vi "T_MXC_control_PK_v1.0.vi"() -> ()   [LabVIEW 2016]
uses:
  Labview Drivers/lake_shore_372/Lake Shore 372/Lake Shore 372.lvlib
panel:
  in  "Output (0: sample heater)":u16(ring) items=["sample heater", "output 1 (warm-up heater) ", "output 2 (analog/still)"]
  in  "Heater Range (0: Off)":u16(ring) items=["Off", "31.6 uA", "100 uA", "316 uA", "1.00 mA", "3.16 mA", "10.0 mA", "31.6 mA", "100 mA"]
  in  "Manual Output (0.000%)":dbl min=-100.0 max=100.0 step=0.001 format="%.3f"
  in  "VISA resource name":refnum<visa-resource-name>="COM3"
  in  "Channel":i32=6
  out "Temperature (K)":dbl=4.98178 format="%#_13g"
  out "Time(s)":dbl=152.218 format="%#_13g"
  out "No. of data points collected":i32=3271
  in  "?":bool
  out "Temperature vs time":cluster{dbl, "Field Reading":dbl}[](graph)=[{0.061, "Field Reading"=5.86421}, {0.103, "Field Reading"=5.86421}, {0.153, "Field Reading"=5.86355}, {0.192, "Field Reading"=5.86355}, {0.254, "Field Reading"=5.86259}, {0.293, "Field Reading"=5.86259}, {0.353, "Field Reading"=5.8614}, {0.394, "Field Reading"=5.8614}, {0.454, "Field Reading"=5.85996}, {0.493, "Field Reading"=5.85996}, {0.549, "Field Reading"=5.85871}, {0.589, "Field Reading"=5.85871}, {0.649, "Field Reading"=5.85721}, {0.688, "Field Reading"=5.85721}, {0.748, "Field Reading"=5.85589}, {0.787, "Field Reading"=5.85589}, {0.826, "Field Reading"=5.8544}, {0.88, "Field Reading"=5.8544}, {0.921, "Field Reading"=5.85278}, {0.98, "Field Reading"=5.85278}, {1.019, "Field Reading"=5.85123}, {1.08, "Field Reading"=5.85123}, {1.121, "Field Reading"=5.84991}, {1.179, "Field Reading"=5.84991}, {1.219, "Field Reading"=5.84991}, {1.269, "Field Reading"=5.8489}, {1.308, "Field Reading"=5.8489}, {1.368, "Field Reading"=5.84782}, {1.405, "Field Reading"=5.84782}, {1.454, "Field Reading"=5.84692}, {1.494, "Field Reading"=5.84692}, {1.555, "Field Reading"=5.84602}, {1.593, "Field Reading"=5.84602}, {1.653, "Field Reading"=5.84537}, {1.694, "Field Reading"=5.84537}, {1.754, "Field Reading"=5.84465}, {1.793, "Field Reading"=5.84465}, {1.854, "Field Reading"=5.84417}, {1.895, "Field Reading"=5.84417}, {1.953, "Field Reading"=5.84351}, {1.994, "Field Reading"=5.84351}, {2.054, "Field Reading"=5.84267}, {2.093, "Field Reading"=5.84267}, {2.152, "Field Reading"=5.84154}, {2.191, "Field Reading"=5.84154}, {2.251, "Field Reading"=5.84022}, {2.29, "Field Reading"=5.84022}, {2.348, "Field Reading"=5.83897}, {2.389, "Field Reading"=5.83897}, {2.449, "Field Reading"=5.83789}, {2.487, "Field Reading"=5.83789}, {2.527, "Field Reading"=5.83693}, {2.58, "Field Reading"=5.83693}, {2.618, "Field Reading"=5.83693}, {2.669, "Field Reading"=5.83603}, {2.707, "Field Reading"=5.83603}, {2.768, "Field Reading"=5.83526}, {2.81, "Field Reading"=5.83526}, {2.867, "Field Reading"=5.83466}, {2.906, "Field Reading"=5.83466}, {2.953, "Field Reading"=5.83394}, {2.992, "Field Reading"=5.83394}, {3.053, "Field Reading"=5.83322}, {3.092, "Field Reading"=5.83322}, {3.153, "Field Reading"=5.83263}, {3.192, "Field Reading"=5.83263}, {3.251, "Field Reading"=5.83179}, {3.29, "Field Reading"=5.83179}, {3.348, "Field Reading"=5.83065}, {3.387, "Field Reading"=5.83065}, {3.425, "Field Reading"=5.82945}, {3.48, "Field Reading"=5.82945}, {3.52, "Field Reading"=5.82945}, {3.569, "Field Reading"=5.82844}, {3.608, "Field Reading"=5.82844}, {3.667, "Field Reading"=5.82718}, {3.707, "Field Reading"=5.82718}, {3.755, "Field Reading"=5.82598}, {3.793, "Field Reading"=5.82598}, {3.857, "Field Reading"=5.82491}, {3.895, "Field Reading"=5.82491}, {3.954, "Field Reading"=5.82365}, {3.992, "Field Reading"=5.82365}, {4.05, "Field Reading"=5.82228}, {4.091, "Field Reading"=5.82228}, {4.149, "Field Reading"=5.82108}, {4.19, "Field Reading"=5.82108}, {4.249, "Field Reading"=5.81988}, {4.288, "Field Reading"=5.81988}, {4.327, "Field Reading"=5.81863}, {4.38, "Field Reading"=5.81863}, {4.421, "Field Reading"=5.81773}, {4.483, "Field Reading"=5.81773}, {4.524, "Field Reading"=5.81677}, {4.583, "Field Reading"=5.81677}, {4.621, "Field Reading"=5.816}, {4.681, "Field Reading"=5.816}, {4.722, "Field Reading"=5.81522}, {4.78, "Field Reading"=5.81522}, {4.819, "Field Reading"=5.81522}, {4.869, "Field Reading"=5.8148}, {4.911, "Field Reading"=5.8148}, {4.968, "Field Reading"=5.81432}, {5.007, "Field Reading"=5.81432}, {5.07, "Field Reading"=5.81384}, {5.109, "Field Reading"=5.81384}, {5.168, "Field Reading"=5.81324}, {5.207, "Field Reading"=5.81324}, {5.269, "Field Reading"=5.81247}, {5.31, "Field Reading"=5.81247}, {5.367, "Field Reading"=5.81205}, {5.406, "Field Reading"=5.81205}, {5.455, "Field Reading"=5.81163}, {5.494, "Field Reading"=5.81163}, {5.555, "Field Reading"=5.81145}, {5.595, "Field Reading"=5.81145}, {5.655, "Field Reading"=5.81091}, {5.694, "Field Reading"=5.81091}, {5.753, "Field Reading"=5.81037}, {5.794, "Field Reading"=5.81037}, {5.852, "Field Reading"=5.80995}, {5.891, "Field Reading"=5.80995}, {5.95, "Field Reading"=5.80954}, {5.988, "Field Reading"=5.80954}, {6.026, "Field Reading"=5.80918}, {6.081, "Field Reading"=5.80918}, {6.12, "Field Reading"=5.80918}, {6.17, "Field Reading"=5.8084}, {6.21, "Field Reading"=5.8084}, {6.27, "Field Reading"=5.80756}, {6.308, "Field Reading"=5.80756}, {6.367, "Field Reading"=5.80654}, {6.406, "Field Reading"=5.80654}, {6.457, "Field Reading"=5.80541}, {6.496, "Field Reading"=5.80541}, {6.554, "Field Reading"=5.80433}, {6.593, "Field Reading"=5.80433}, {6.652, "Field Reading"=5.80331}, {6.691, "Field Reading"=5.80331}, {6.751, "Field Reading"=5.8023}, {6.793, "Field Reading"=5.8023}, {6.851, "Field Reading"=5.80116}, {6.892, "Field Reading"=5.80116}, {6.949, "Field Reading"=5.80026}, {6.987, "Field Reading"=5.80026}, {7.029, "Field Reading"=5.79913}, {7.082, "Field Reading"=5.79913}, {7.122, "Field Reading"=5.79829}, {7.182, "Field Reading"=5.79829}, {7.223, "Field Reading"=5.79781}, {7.283, "Field Reading"=5.79781}, {7.324, "Field Reading"=5.79739}, {7.383, "Field Reading"=5.79739}, {7.422, "Field Reading"=5.79715}, {7.483, "Field Reading"=5.79715}, {7.523, "Field Reading"=5.79662}, {7.584, "Field Reading"=5.79662}, {7.625, "Field Reading"=5.79638}, {7.681, "Field Reading"=5.79638}, {7.722, "Field Reading"=5.7959}, {7.782, "Field Reading"=5.7959}, {7.824, "Field Reading"=5.7956}, {7.882, "Field Reading"=5.7956}, {7.921, "Field Reading"=5.7956}, {7.969, "Field Reading"=5.7947}, {8.008, "Field Reading"=5.7947}, {8.069, "Field Reading"=5.79374}, {8.107, "Field Reading"=5.79374}, {8.168, "Field Reading"=5.79255}, {8.208, "Field Reading"=5.79255}, {8.256, "Field Reading"=5.79111}, {8.297, "Field Reading"=5.79111}, {8.354, "Field Reading"=5.78962}, {8.393, "Field Reading"=5.78962}, {8.451, "Field Reading"=5.78794}, {8.492, "Field Reading"=5.78794}, {8.549, "Field Reading"=5.78627}, {8.59, "Field Reading"=5.78627}, {8.651, "Field Reading"=5.78447}, {8.691, "Field Reading"=5.78447}, {8.749, "Field Reading"=5.78286}, {8.789, "Field Reading"=5.78286}, {8.827, "Field Reading"=5.7813}, {8.882, "Field Reading"=5.7813}, {8.921, "Field Reading"=5.7813}, {8.969, "Field Reading"=5.77993}, {9.008, "Field Reading"=5.77993}, {9.056, "Field Reading"=5.77861}, {9.095, "Field Reading"=5.77861}, {9.157, "Field Reading"=5.77753}, {9.196, "Field Reading"=5.77753}, {9.257, "Field Reading"=5.7764}, {9.3, "Field Reading"=5.7764}, {9.356, "Field Reading"=5.77544}, {9.395, "Field Reading"=5.77544}, {9.457, "Field Reading"=5.77418}, {9.498, "Field Reading"=5.77418}, {9.555, "Field Reading"=5.77287}, {9.595, "Field Reading"=5.77287}, {9.653, "Field Reading"=5.77137}, {9.695, "Field Reading"=5.77137}, {9.755, "Field Reading"=5.77018}, {9.794, "Field Reading"=5.77018}, {9.852, "Field Reading"=5.76886}, {9.89, "Field Reading"=5.76886}, {9.95, "Field Reading"=5.76736}, {9.99, "Field Reading"=5.76736}, {10.029, "Field Reading"=5.76599}, {10.084, "Field Reading"=5.76599}, {10.125, "Field Reading"=5.76455}, {10.182, "Field Reading"=5.76455}, {10.222, "Field Reading"=5.76455}, {10.271, "Field Reading"=5.76342}, {10.31, "Field Reading"=5.76342}, {10.369, "Field Reading"=5.76252}, {10.41, "Field Reading"=5.76252}, {10.47, "Field Reading"=5.76162}, {10.51, "Field Reading"=5.76162}, {10.569, "Field Reading"=5.76019}, {10.608, "Field Reading"=5.76019}, {10.67, "Field Reading"=5.75911}, {10.711, "Field Reading"=5.75911}, {10.77, "Field Reading"=5.75827}, {10.808, "Field Reading"=5.75827}, {10.856, "Field Reading"=5.75761}, {10.895, "Field Reading"=5.75761}, {10.955, "Field Reading"=5.75714}, {10.995, "Field Reading"=5.75714}, {11.056, "Field Reading"=5.75672}, {11.096, "Field Reading"=5.75672}, {11.155, "Field Reading"=5.75618}, {11.195, "Field Reading"=5.75618}, {11.253, "Field Reading"=5.75552}, {11.291, "Field Reading"=5.75552}, {11.351, "Field Reading"=5.75504}, {11.39, "Field Reading"=5.75504}, {11.429, "Field Reading"=5.75426}, {11.483, "Field Reading"=5.75426}, {11.524, "Field Reading"=5.75343}, {11.581, "Field Reading"=5.75343}, {11.621, "Field Reading"=5.75343}, {11.672, "Field Reading"=5.75235}, {11.711, "Field Reading"=5.75235}, {11.769, "Field Reading"=5.75121}, {11.809, "Field Reading"=5.75121}, {11.858, "Field Reading"=5.74996}, {11.899, "Field Reading"=5.74996}, {11.955, "Field Reading"=5.7487}, {11.996, "Field Reading"=5.7487}, {12.058, "Field Reading"=5.74757}, {12.098, "Field Reading"=5.74757}, {12.155, "Field Reading"=5.74643}, {12.196, "Field Reading"=5.74643}, {12.256, "Field Reading"=5.74565}, {12.296, "Field Reading"=5.74565}, {12.355, "Field Reading"=5.74463}, {12.394, "Field Reading"=5.74463}, {12.452, "Field Reading"=5.74374}, {12.491, "Field Reading"=5.74374}, {12.551, "Field Reading"=5.74266}, {12.592, "Field Reading"=5.74266}, {12.652, "Field Reading"=5.7417}, {12.692, "Field Reading"=5.7417}, {12.751, "Field Reading"=5.74087}, {12.79, "Field Reading"=5.74087}, {12.852, "Field Reading"=5.73991}, {12.89, "Field Reading"=5.73991}, {12.93, "Field Reading"=5.73877}, {12.985, "Field Reading"=5.73877}, {13.024, "Field Reading"=5.7374}, {13.087, "Field Reading"=5.7374}, {13.125, "Field Reading"=5.7362}, {13.184, "Field Reading"=5.7362}, {13.222, "Field Reading"=5.73464}, {13.283, "Field Reading"=5.73464}, {13.322, "Field Reading"=5.73464}, {13.37, "Field Reading"=5.73327}, {13.409, "Field Reading"=5.73327}, {13.457, "Field Reading"=5.73183}, {13.496, "Field Reading"=5.73183}, {13.553, "Field Reading"=5.7304}, {13.592, "Field Reading"=5.7304}, {13.651, "Field Reading"=5.72908}, {13.692, "Field Reading"=5.72908}, {13.751, "Field Reading"=5.72795}, {13.791, "Field Reading"=5.72795}, {13.829, "Field Reading"=5.72693}, {13.884, "Field Reading"=5.72693}, {13.926, "Field Reading"=5.72579}, {13.982, "Field Reading"=5.72579}, {14.021, "Field Reading"=5.72579}, {14.071, "Field Reading"=5.72501}, {14.111, "Field Reading"=5.72501}, {14.169, "Field Reading"=5.72388}, {14.207, "Field Reading"=5.72388}, {14.259, "Field Reading"=5.72256}, {14.298, "Field Reading"=5.72256}, {14.356, "Field Reading"=5.72113}, {14.398, "Field Reading"=5.72113}, {14.457, "Field Reading"=5.71951}, {14.495, "Field Reading"=5.71951}, {14.552, "Field Reading"=5.71778}, {14.591, "Field Reading"=5.71778}, {14.652, "Field Reading"=5.7158}, {14.693, "Field Reading"=5.7158}, {14.751, "Field Reading"=5.71401}, {14.79, "Field Reading"=5.71401}, {14.852, "Field Reading"=5.71209}, {14.89, "Field Reading"=5.71209}, {14.929, "Field Reading"=5.71078}, {14.985, "Field Reading"=5.71078}, {15.024, "Field Reading"=5.7093}, {15.083, "Field Reading"=5.7093}, {15.124, "Field Reading"=5.70789}, {15.183, "Field Reading"=5.70789}, {15.223, "Field Reading"=5.70657}, {15.283, "Field Reading"=5.70657}, {15.323, "Field Reading"=5.70541}, {15.385, "Field Reading"=5.70541}, {15.423, "Field Reading"=5.70448}, {15.486, "Field Reading"=5.70448}, {15.526, "Field Reading"=5.70358}, {15.582, "Field Reading"=5.70358}, {15.621, "Field Reading"=5.70358}, {15.672, "Field Reading"=5.70281}, {15.712, "Field Reading"=5.70281}, {15.77, "Field Reading"=5.70197}, {15.812, "Field Reading"=5.70197}, {15.87, "Field Reading"=5.70116}, {15.911, "Field Reading"=5.70116}, {15.97, "Field Reading"=5.70035}, {16.009, "Field Reading"=5.70035}, {16.058, "Field Reading"=5.69937}, {16.098, "Field Reading"=5.69937}, {16.156, "Field Reading"=5.69859}, {16.197, "Field Reading"=5.69859}, {16.255, "Field Reading"=5.69751}, {16.297, "Field Reading"=5.69751}, {16.358, "Field Reading"=5.69643}, {16.398, "Field Reading"=5.69643}, {16.458, "Field Reading"=5.6953}, {16.498, "Field Reading"=5.6953}, {16.556, "Field Reading"=5.69416}, {16.595, "Field Reading"=5.69416}, {16.655, "Field Reading"=5.69317}, {16.695, "Field Reading"=5.69317}, {16.752, "Field Reading"=5.69204}, {16.79, "Field Reading"=5.69204}, {16.829, "Field Reading"=5.69093}, {16.886, "Field Reading"=5.69093}, {16.925, "Field Reading"=5.68964}, {16.983, "Field Reading"=5.68964}, {17.022, "Field Reading"=5.68964}, {17.075, "Field Reading"=5.68845}, {17.115, "Field Reading"=5.68845}, {17.171, "Field Reading"=5.68743}, {17.21, "Field Reading"=5.68743}, {17.258, "Field Reading"=5.68647}, {17.299, "Field Reading"=5.68647}, {17.355, "Field Reading"=5.68513}, {17.395, "Field Reading"=5.68513}, {17.45, "Field Reading"=5.68399}, {17.489, "Field Reading"=5.68399}, {17.528, "Field Reading"=5.68327}, {17.583, "Field Reading"=5.68327}, {17.622, "Field Reading"=5.68327}, {17.669, "Field Reading"=5.68271}, {17.712, "Field Reading"=5.68271}, {17.769, "Field Reading"=5.68214}, {17.808, "Field Reading"=5.68214}, {17.856, "Field Reading"=5.68175}, {17.896, "Field Reading"=5.68175}, {17.952, "Field Reading"=5.68103}, {17.993, "Field Reading"=5.68103}, {18.031, "Field Reading"=5.68028}, {18.082, "Field Reading"=5.68028}, {18.122, "Field Reading"=5.68028}, {18.169, "Field Reading"=5.67986}, {18.208, "Field Reading"=5.67986}, {18.255, "Field Reading"=5.67956}, {18.296, "Field Reading"=5.67956}, {18.351, "Field Reading"=5.67912}, {18.389, "Field Reading"=5.67912}, {18.428, "Field Reading"=5.6787}, {18.484, "Field Reading"=5.6787}, {18.523, "Field Reading"=5.6787}, {18.571, "Field Reading"=5.6781}, {18.612, "Field Reading"=5.6781}, {18.669, "Field Reading"=5.6775}, {18.708, "Field Reading"=5.6775}, {18.755, "Field Reading"=5.67717}, {18.796, "Field Reading"=5.67717}, {18.853, "Field Reading"=5.67669}, {18.893, "Field Reading"=5.67669}, {18.95, "Field Reading"=5.67624}, {18.989, "Field Reading"=5.67624}, {19.03, "Field Reading"=5.67562}, {19.082, "Field Reading"=5.67562}, {19.123, "Field Reading"=5.67562}, {19.169, "Field Reading"=5.67481}, {19.208, "Field Reading"=5.67481}, {19.258, "Field Reading"=5.6737}, {19.297, "Field Reading"=5.6737}, {19.355, "Field Reading"=5.67254}, {19.393, "Field Reading"=5.67254}, {19.451, "Field Reading"=5.6711}, {19.491, "Field Reading"=5.6711}, {19.551, "Field Reading"=5.66972}, {19.589, "Field Reading"=5.66972}, {19.627, "Field Reading"=5.66847}, {19.683, "Field Reading"=5.66847}, {19.722, "Field Reading"=5.66847}, {19.77, "Field Reading"=5.66718}, {19.812, "Field Reading"=5.66718}, {19.868, "Field Reading"=5.6659}, {19.91, "Field Reading"=5.6659}, {19.957, "Field Reading"=5.66464}, {19.997, "Field Reading"=5.66464}, {20.056, "Field Reading"=5.66365}, {20.095, "Field Reading"=5.66365}, {20.15, "Field Reading"=5.66296}, {20.189, "Field Reading"=5.66296}, {20.227, "Field Reading"=5.66243}, {20.282, "Field Reading"=5.66243}, {20.321, "Field Reading"=5.66243}, {20.369, "Field Reading"=5.66192}, {20.41, "Field Reading"=5.66192}, {20.458, "Field Reading"=5.66132}, {20.496, "Field Reading"=5.66132}, {20.552, "Field Reading"=5.66066}, {20.59, "Field Reading"=5.66066}, {20.628, "Field Reading"=5.66021}, {20.683, "Field Reading"=5.66021}, {20.723, "Field Reading"=5.66021}, {20.77, "Field Reading"=5.65967}, {20.808, "Field Reading"=5.65967}, {20.856, "Field Reading"=5.65908}, {20.896, "Field Reading"=5.65908}, {20.952, "Field Reading"=5.65848}, {20.992, "Field Reading"=5.65848}, {21.032, "Field Reading"=5.65791}, {21.082, "Field Reading"=5.65791}, {21.121, "Field Reading"=5.65791}, {21.169, "Field Reading"=5.65737}, {21.207, "Field Reading"=5.65737}, {21.257, "Field Reading"=5.65683}, {21.296, "Field Reading"=5.65683}, {21.351, "Field Reading"=5.65626}, {21.392, "Field Reading"=5.65626}, {21.43, "Field Reading"=5.6557}, {21.483, "Field Reading"=5.6557}, {21.524, "Field Reading"=5.6557}, {21.57, "Field Reading"=5.65519}, {21.609, "Field Reading"=5.65519}, {21.657, "Field Reading"=5.65471}, {21.698, "Field Reading"=5.65471}, {21.756, "Field Reading"=5.65426}, {21.796, "Field Reading"=5.65426}, {21.853, "Field Reading"=5.65378}, {21.891, "Field Reading"=5.65378}, {21.929, "Field Reading"=5.65309}, {21.981, "Field Reading"=5.65309}, {22.021, "Field Reading"=5.65309}, {22.07, "Field Reading"=5.65259}, {22.109, "Field Reading"=5.65259}, {22.156, "Field Reading"=5.65205}, {22.196, "Field Reading"=5.65205}, {22.252, "Field Reading"=5.6513}, {22.292, "Field Reading"=5.6513}, {22.331, "Field Reading"=5.65034}, {22.382, "Field Reading"=5.65034}, {22.421, "Field Reading"=5.65034}, {22.47, "Field Reading"=5.64926}, {22.508, "Field Reading"=5.64926}, {22.556, "Field Reading"=5.64825}, {22.594, "Field Reading"=5.64825}, {22.651, "Field Reading"=5.6472}, {22.691, "Field Reading"=5.6472}, {22.73, "Field Reading"=5.64618}, {22.781, "Field Reading"=5.64618}, {22.82, "Field Reading"=5.64618}, {22.87, "Field Reading"=5.64526}, {22.908, "Field Reading"=5.64526}, {22.956, "Field Reading"=5.64442}, {22.994, "Field Reading"=5.64442}, {23.052, "Field Reading"=5.64379}, {23.093, "Field Reading"=5.64379}, {23.151, "Field Reading"=5.64316}, {23.191, "Field Reading"=5.64316}, {23.231, "Field Reading"=5.6428}, {23.283, "Field Reading"=5.6428}, {23.323, "Field Reading"=5.6428}, {23.37, "Field Reading"=5.64242}, {23.409, "Field Reading"=5.64242}, {23.457, "Field Reading"=5.64206}, {23.496, "Field Reading"=5.64206}, {23.551, "Field Reading"=5.64158}, {23.592, "Field Reading"=5.64158}, {23.652, "Field Reading"=5.6411}, {23.691, "Field Reading"=5.6411}, {23.73, "Field Reading"=5.64071}, {23.781, "Field Reading"=5.64071}, {23.821, "Field Reading"=5.64071}, {23.87, "Field Reading"=5.64032}, {23.908, "Field Reading"=5.64032}, {23.957, "Field Reading"=5.6402}, {23.998, "Field Reading"=5.6402}, {24.058, "Field Reading"=5.64017}, {24.098, "Field Reading"=5.64017}, {24.157, "Field Reading"=5.63996}, {24.197, "Field Reading"=5.63996}, {24.253, "Field Reading"=5.63948}, {24.293, "Field Reading"=5.63948}, {24.332, "Field Reading"=5.63933}, {24.384, "Field Reading"=5.63933}, {24.422, "Field Reading"=5.63933}, {24.471, "Field Reading"=5.63883}, {24.511, "Field Reading"=5.63883}, {24.556, "Field Reading"=5.6382}, {24.597, "Field Reading"=5.6382}, {24.654, "Field Reading"=5.63715}, {24.695, "Field Reading"=5.63715}, {24.751, "Field Reading"=5.63604}, {24.79, "Field Reading"=5.63604}, {24.828, "Field Reading"=5.63464}, {24.883, "Field Reading"=5.63464}, {24.922, "Field Reading"=5.63464}, {24.97, "Field Reading"=5.63332}, {25.012, "Field Reading"=5.63332}, {25.059, "Field Reading"=5.63231}, {25.099, "Field Reading"=5.63231}, {25.153, "Field Reading"=5.63114}, {25.195, "Field Reading"=5.63114}, {25.252, "Field Reading"=5.63}, {25.292, "Field Reading"=5.63}, {25.333, "Field Reading"=5.62872}, {25.382, "Field Reading"=5.62872}, {25.422, "Field Reading"=5.62872}, {25.471, "Field Reading"=5.62752}, {25.511, "Field Reading"=5.62752}, {25.557, "Field Reading"=5.62626}, {25.595, "Field Reading"=5.62626}, {25.652, "Field Reading"=5.62501}, {25.691, "Field Reading"=5.62501}, {25.731, "Field Reading"=5.62354}, {25.787, "Field Reading"=5.62354}, {25.828, "Field Reading"=5.62205}, {25.883, "Field Reading"=5.62205}, {25.923, "Field Reading"=5.62205}, {25.97, "Field Reading"=5.62049}, {26.008, "Field Reading"=5.62049}, {26.057, "Field Reading"=5.61899}, {26.097, "Field Reading"=5.61899}, {26.153, "Field Reading"=5.61756}, {26.192, "Field Reading"=5.61756}, {26.233, "Field Reading"=5.61663}, {26.284, "Field Reading"=5.61663}, {26.323, "Field Reading"=5.61663}, {26.371, "Field Reading"=5.6157}, {26.41, "Field Reading"=5.6157}, {26.459, "Field Reading"=5.61481}, {26.499, "Field Reading"=5.61481}, {26.554, "Field Reading"=5.61379}, {26.592, "Field Reading"=5.61379}, {26.632, "Field Reading"=5.61271}, {26.685, "Field Reading"=5.61271}, {26.724, "Field Reading"=5.61271}, {26.771, "Field Reading"=5.61152}, {26.812, "Field Reading"=5.61152}, {26.858, "Field Reading"=5.61032}, {26.899, "Field Reading"=5.61032}, {26.953, "Field Reading"=5.60906}, {26.992, "Field Reading"=5.60906}, {27.032, "Field Reading"=5.60745}, {27.086, "Field Reading"=5.60745}, {27.125, "Field Reading"=5.60745}, {27.172, "Field Reading"=5.60565}, {27.212, "Field Reading"=5.60565}, {27.258, "Field Reading"=5.60404}, {27.296, "Field Reading"=5.60404}, {27.353, "Field Reading"=5.6026}, {27.393, "Field Reading"=5.6026}, {27.453, "Field Reading"=5.60114}, {27.492, "Field Reading"=5.60114}, {27.531, "Field Reading"=5.59988}, {27.586, "Field Reading"=5.59988}, {27.625, "Field Reading"=5.59988}, {27.673, "Field Reading"=5.59857}, {27.715, "Field Reading"=5.59857}, {27.771, "Field Reading"=5.59725}, {27.812, "Field Reading"=5.59725}, {27.859, "Field Reading"=5.59599}, {27.897, "Field Reading"=5.59599}, {27.954, "Field Reading"=5.59498}, {27.992, "Field Reading"=5.59498}, {28.033, "Field Reading"=5.59387}, {28.086, "Field Reading"=5.59387}, {28.124, "Field Reading"=5.59387}, {28.171, "Field Reading"=5.59267}, {28.211, "Field Reading"=5.59267}, {28.258, "Field Reading"=5.59157}, {28.296, "Field Reading"=5.59157}, {28.352, "Field Reading"=5.59046}, {28.393, "Field Reading"=5.59046}, {28.432, "Field Reading"=5.58941}, {28.485, "Field Reading"=5.58941}, {28.523, "Field Reading"=5.58941}, {28.57, "Field Reading"=5.58854}, {28.611, "Field Reading"=5.58854}, {28.659, "Field Reading"=5.58768}, {28.699, "Field Reading"=5.58768}, {28.754, "Field Reading"=5.58663}, {28.793, "Field Reading"=5.58663}, {28.831, "Field Reading"=5.58558}, {28.885, "Field Reading"=5.58558}, {28.926, "Field Reading"=5.58558}, {28.971, "Field Reading"=5.58487}, {29.01, "Field Reading"=5.58487}, {29.06, "Field Reading"=5.58412}, {29.099, "Field Reading"=5.58412}, {29.155, "Field Reading"=5.58337}, {29.196, "Field Reading"=5.58337}, {29.254, "Field Reading"=5.5828}, {29.293, "Field Reading"=5.5828}, {29.332, "Field Reading"=5.5822}, {29.384, "Field Reading"=5.5822}, {29.423, "Field Reading"=5.5822}, {29.471, "Field Reading"=5.58184}, {29.51, "Field Reading"=5.58184}, {29.558, "Field Reading"=5.58149}, {29.597, "Field Reading"=5.58149}, {29.654, "Field Reading"=5.58119}, {29.691, "Field Reading"=5.58119}, {29.732, "Field Reading"=5.58065}, {29.786, "Field Reading"=5.58065}, {29.824, "Field Reading"=5.58065}, {29.872, "Field Reading"=5.58008}, {29.911, "Field Reading"=5.58008}, {29.957, "Field Reading"=5.5796}, {29.998, "Field Reading"=5.5796}, {30.054, "Field Reading"=5.57903}, {30.093, "Field Reading"=5.57903}, {30.133, "Field Reading"=5.57829}, {30.184, "Field Reading"=5.57829}, {30.223, "Field Reading"=5.57829}, {30.272, "Field Reading"=5.57736}, {30.312, "Field Reading"=5.57736}, {30.358, "Field Reading"=5.57637}, {30.397, "Field Reading"=5.57637}, {30.454, "Field Reading"=5.57532}, {30.493, "Field Reading"=5.57532}, {30.53, "Field Reading"=5.57434}, {30.586, "Field Reading"=5.57434}, {30.625, "Field Reading"=5.57434}, {30.674, "Field Reading"=5.57332}, {30.715, "Field Reading"=5.57332}, {30.771, "Field Reading"=5.57212}, {30.811, "Field Reading"=5.57212}, {30.859, "Field Reading"=5.57072}, {30.897, "Field Reading"=5.57072}, {30.953, "Field Reading"=5.5694}, {30.993, "Field Reading"=5.5694}, {31.031, "Field Reading"=5.56785}, {31.086, "Field Reading"=5.56785}, {31.127, "Field Reading"=5.56647}, {31.185, "Field Reading"=5.56647}, {31.226, "Field Reading"=5.56647}, {31.274, "Field Reading"=5.56521}, {31.313, "Field Reading"=5.56521}, {31.371, "Field Reading"=5.5639}, {31.41, "Field Reading"=5.5639}, {31.46, "Field Reading"=5.56276}, {31.5, "Field Reading"=5.56276}, {31.555, "Field Reading"=5.56168}, {31.594, "Field Reading"=5.56168}, {31.633, "Field Reading"=5.56088}, {31.686, "Field Reading"=5.56088}, {31.726, "Field Reading"=5.56088}, {31.772, "Field Reading"=5.56004}, {31.813, "Field Reading"=5.56004}, {31.859, "Field Reading"=5.55935}, {31.9, "Field Reading"=5.55935}, {31.954, "Field Reading"=5.55875}, {31.992, "Field Reading"=5.55875}, {32.032, "Field Reading"=5.5578}, {32.085, "Field Reading"=5.5578}, {32.124, "Field Reading"=5.5578}, {32.171, "Field Reading"=5.55696}, {32.211, "Field Reading"=5.55696}, {32.259, "Field Reading"=5.55618}, {32.297, "Field Reading"=5.55618}, {32.353, "Field Reading"=5.55552}, {32.391, "Field Reading"=5.55552}, {32.43, "Field Reading"=5.55486}, {32.485, "Field Reading"=5.55486}, {32.525, "Field Reading"=5.55486}, {32.571, "Field Reading"=5.55427}, {32.613, "Field Reading"=5.55427}, {32.66, "Field Reading"=5.55391}, {32.699, "Field Reading"=5.55391}, {32.754, "Field Reading"=5.5537}, {32.793, "Field Reading"=5.5537}, {32.831, "Field Reading"=5.55367}, {32.886, "Field Reading"=5.55367}, {32.924, "Field Reading"=5.55367}, {32.973, "Field Reading"=5.55352}, {33.013, "Field Reading"=5.55352}, {33.06, "Field Reading"=5.55322}, {33.098, "Field Reading"=5.55322}, {33.154, "Field Reading"=5.55295}, {33.193, "Field Reading"=5.55295}, {33.232, "Field Reading"=5.55229}, {33.286, "Field Reading"=5.55229}, {33.327, "Field Reading"=5.55157}, {33.385, "Field Reading"=5.55157}, {33.423, "Field Reading"=5.55157}, {33.473, "Field Reading"=5.55071}, {33.513, "Field Reading"=5.55071}, {33.558, "Field Reading"=5.5499}, {33.598, "Field Reading"=5.5499}, {33.655, "Field Reading"=5.549}, {33.693, "Field Reading"=5.549}, {33.734, "Field Reading"=5.54831}, {33.784, "Field Reading"=5.54831}, {33.824, "Field Reading"=5.54831}, {33.874, "Field Reading"=5.54781}, {33.913, "Field Reading"=5.54781}, {33.959, "Field Reading"=5.54739}, {33.997, "Field Reading"=5.54739}, {34.055, "Field Reading"=5.54718}, {34.094, "Field Reading"=5.54718}, {34.134, "Field Reading"=5.54697}, {34.187, "Field Reading"=5.54697}, {34.227, "Field Reading"=5.54697}, {34.274, "Field Reading"=5.54673}, {34.315, "Field Reading"=5.54673}, {34.359, "Field Reading"=5.54619}, {34.399, "Field Reading"=5.54619}, {34.456, "Field Reading"=5.5458}, {34.496, "Field Reading"=5.5458}, {34.535, "Field Reading"=5.54526}, {34.585, "Field Reading"=5.54526}, {34.625, "Field Reading"=5.54526}, {34.675, "Field Reading"=5.54452}, {34.713, "Field Reading"=5.54452}, {34.759, "Field Reading"=5.54377}, {34.797, "Field Reading"=5.54377}, {34.855, "Field Reading"=5.54302}, {34.895, "Field Reading"=5.54302}, {34.954, "Field Reading"=5.54218}, {34.992, "Field Reading"=5.54218}, {35.032, "Field Reading"=5.54138}, {35.086, "Field Reading"=5.54138}, {35.125, "Field Reading"=5.54138}, {35.172, "Field Reading"=5.54075}, {35.211, "Field Reading"=5.54075}, {35.26, "Field Reading"=5.54024}, {35.299, "Field Reading"=5.54024}, {35.355, "Field Reading"=5.53966}, {35.394, "Field Reading"=5.53966}, {35.434, "Field Reading"=5.5391}, {35.486, "Field Reading"=5.5391}, {35.525, "Field Reading"=5.5391}, {35.572, "Field Reading"=5.53832}, {35.612, "Field Reading"=5.53832}, {35.659, "Field Reading"=5.53776}, {35.699, "Field Reading"=5.53776}, {35.754, "Field Reading"=5.53731}, {35.793, "Field Reading"=5.53731}, {35.832, "Field Reading"=5.53686}, {35.886, "Field Reading"=5.53686}, {35.925, "Field Reading"=5.53686}, {35.972, "Field Reading"=5.5363}, {36.011, "Field Reading"=5.5363}, {36.06, "Field Reading"=5.53557}, {36.1, "Field Reading"=5.53557}, {36.156, "Field Reading"=5.53495}, {36.196, "Field Reading"=5.53495}, {36.234, "Field Reading"=5.53422}, {36.286, "Field Reading"=5.53422}, {36.327, "Field Reading"=5.53422}, {36.374, "Field Reading"=5.53344}, {36.415, "Field Reading"=5.53344}, {36.474, "Field Reading"=5.53248}, {36.515, "Field Reading"=5.53248}, {36.56, "Field Reading"=5.53164}, {36.598, "Field Reading"=5.53164}, {36.655, "Field Reading"=5.53052}, {36.696, "Field Reading"=5.53052}, {36.755, "Field Reading"=5.52956}, {36.793, "Field Reading"=5.52956}, {36.832, "Field Reading"=5.52861}, {36.887, "Field Reading"=5.52861}, {36.926, "Field Reading"=5.52861}, {36.974, "Field Reading"=5.52755}, {37.012, "Field Reading"=5.52755}, {37.061, "Field Reading"=5.52654}, {37.099, "Field Reading"=5.52654}, {37.155, "Field Reading"=5.52581}, {37.195, "Field Reading"=5.52581}, {37.235, "Field Reading"=5.52508}, {37.287, "Field Reading"=5.52508}, {37.326, "Field Reading"=5.52508}, {37.374, "Field Reading"=5.52435}, {37.412, "Field Reading"=5.52435}, {37.462, "Field Reading"=5.52379}, {37.501, "Field Reading"=5.52379}, {37.556, "Field Reading"=5.52334}, {37.596, "Field Reading"=5.52334}, {37.656, "Field Reading"=5.52272}, {37.697, "Field Reading"=5.52272}, {37.735, "Field Reading"=5.52205}, {37.785, "Field Reading"=5.52205}, {37.824, "Field Reading"=5.52205}, {37.873, "Field Reading"=5.52132}, {37.912, "Field Reading"=5.52132}, {37.959, "Field Reading"=5.52042}, {38.001, "Field Reading"=5.52042}, {38.06, "Field Reading"=5.51958}, {38.101, "Field Reading"=5.51958}, {38.156, "Field Reading"=5.51868}, {38.195, "Field Reading"=5.51868}, {38.234, "Field Reading"=5.5179}, {38.286, "Field Reading"=5.5179}, {38.327, "Field Reading"=5.5179}, {38.375, "Field Reading"=5.51694}, {38.414, "Field Reading"=5.51694}, {38.461, "Field Reading"=5.5161}, {38.499, "Field Reading"=5.5161}, {38.555, "Field Reading"=5.51532}, {38.594, "Field Reading"=5.51532}, {38.633, "Field Reading"=5.51459}, {38.687, "Field Reading"=5.51459}, {38.727, "Field Reading"=5.51459}, {38.773, "Field Reading"=5.51397}, {38.813, "Field Reading"=5.51397}, {38.862, "Field Reading"=5.5133}, {38.902, "Field Reading"=5.5133}, {38.957, "Field Reading"=5.5124}, {38.996, "Field Reading"=5.5124}, {39.035, "Field Reading"=5.5115}, {39.087, "Field Reading"=5.5115}, {39.126, "Field Reading"=5.5115}, {39.173, "Field Reading"=5.51055}, {39.213, "Field Reading"=5.51055}, {39.26, "Field Reading"=5.50931}, {39.301, "Field Reading"=5.50931}, {39.356, "Field Reading"=5.50819}, {39.395, "Field Reading"=5.50819}, {39.435, "Field Reading"=5.50724}, {39.487, "Field Reading"=5.50724}, {39.527, "Field Reading"=5.50724}, {39.574, "Field Reading"=5.50628}, {39.614, "Field Reading"=5.50628}, {39.663, "Field Reading"=5.5051}, {39.702, "Field Reading"=5.5051}, {39.761, "Field Reading"=5.50387}, {39.802, "Field Reading"=5.50387}, {39.861, "Field Reading"=5.50269}, {39.902, "Field Reading"=5.50269}, {39.957, "Field Reading"=5.50163}, {39.996, "Field Reading"=5.50163}, {40.036, "Field Reading"=5.50079}, {40.088, "Field Reading"=5.50079}, {40.126, "Field Reading"=5.50079}, {40.173, "Field Reading"=5.49978}, {40.213, "Field Reading"=5.49978}, {40.263, "Field Reading"=5.49877}, {40.303, "Field Reading"=5.49877}, {40.357, "Field Reading"=5.49792}, {40.398, "Field Reading"=5.49792}, {40.435, "Field Reading"=5.4972}, {40.488, "Field Reading"=5.4972}, {40.527, "Field Reading"=5.4972}, {40.574, "Field Reading"=5.49647}, {40.613, "Field Reading"=5.49647}, {40.661, "Field Reading"=5.49574}, {40.702, "Field Reading"=5.49574}, {40.758, "Field Reading"=5.49495}, {40.797, "Field Reading"=5.49495}, {40.836, "Field Reading"=5.49422}, {40.887, "Field Reading"=5.49422}, {40.926, "Field Reading"=5.49422}, {40.974, "Field Reading"=5.4936}, {41.016, "Field Reading"=5.4936}, {41.076, "Field Reading"=5.49299}, {41.114, "Field Reading"=5.49299}, {41.16, "Field Reading"=5.49243}, {41.2, "Field Reading"=5.49243}, {41.257, "Field Reading"=5.49198}, {41.296, "Field Reading"=5.49198}, {41.337, "Field Reading"=5.49164}, {41.388, "Field Reading"=5.49164}, {41.426, "Field Reading"=5.49164}, {41.474, "Field Reading"=5.49136}, {41.513, "Field Reading"=5.49136}, {41.56, "Field Reading"=5.49102}, {41.601, "Field Reading"=5.49102}, {41.656, "Field Reading"=5.49052}, {41.696, "Field Reading"=5.49052}, {41.736, "Field Reading"=5.48996}, {41.786, "Field Reading"=5.48996}, {41.825, "Field Reading"=5.48996}, {41.876, "Field Reading"=5.48923}, {41.916, "Field Reading"=5.48923}, {41.974, "Field Reading"=5.48827}, {42.015, "Field Reading"=5.48827}, {42.063, "Field Reading"=5.4871}, {42.104, "Field Reading"=5.4871}, {42.159, "Field Reading"=5.48575}, {42.196, "Field Reading"=5.48575}, {42.257, "Field Reading"=5.48429}, {42.295, "Field Reading"=5.48429}, {42.336, "Field Reading"=5.48289}, {42.387, "Field Reading"=5.48289}, {42.426, "Field Reading"=5.48289}, {42.476, "Field Reading"=5.48149}, {42.516, "Field Reading"=5.48149}, {42.562, "Field Reading"=5.48014}, {42.602, "Field Reading"=5.48014}, {42.658, "Field Reading"=5.47891}, {42.699, "Field Reading"=5.47891}, {42.755, "Field Reading"=5.47778}, {42.796, "Field Reading"=5.47778}, {42.835, "Field Reading"=5.47672}, {42.887, "Field Reading"=5.47672}, {42.926, "Field Reading"=5.47672}, {42.975, "Field Reading"=5.47571}, {43.016, "Field Reading"=5.47571}, {43.062, "Field Reading"=5.47487}, {43.101, "Field Reading"=5.47487}, {43.156, "Field Reading"=5.47403}, {43.196, "Field Reading"=5.47403}, {43.234, "Field Reading"=5.47335}, {43.288, "Field Reading"=5.47335}, {43.328, "Field Reading"=5.47335}, {43.375, "Field Reading"=5.47274}, {43.415, "Field Reading"=5.47274}, {43.463, "Field Reading"=5.47206}, {43.501, "Field Reading"=5.47206}, {43.557, "Field Reading"=5.47122}, {43.595, "Field Reading"=5.47122}, {43.633, "Field Reading"=5.47066}, {43.688, "Field Reading"=5.47066}, {43.726, "Field Reading"=5.47066}, {43.774, "Field Reading"=5.47004}, {43.813, "Field Reading"=5.47004}, {43.864, "Field Reading"=5.46943}, {43.904, "Field Reading"=5.46943}, {43.959, "Field Reading"=5.46864}, {43.998, "Field Reading"=5.46864}, {44.036, "Field Reading"=5.46763}, {44.09, "Field Reading"=5.46763}, {44.129, "Field Reading"=5.46763}, {44.175, "Field Reading"=5.46662}, {44.215, "Field Reading"=5.46662}, {44.262, "Field Reading"=5.46572}, {44.302, "Field Reading"=5.46572}, {44.359, "Field Reading"=5.46482}, {44.399, "Field Reading"=5.46482}, {44.438, "Field Reading"=5.46381}, {44.488, "Field Reading"=5.46381}, {44.526, "Field Reading"=5.46381}, {44.574, "Field Reading"=5.46286}, {44.614, "Field Reading"=5.46286}, {44.663, "Field Reading"=5.46202}, {44.703, "Field Reading"=5.46202}, {44.757, "Field Reading"=5.46123}, {44.796, "Field Reading"=5.46123}, {44.836, "Field Reading"=5.46079}, {44.889, "Field Reading"=5.46079}, {44.929, "Field Reading"=5.46079}, {44.976, "Field Reading"=5.46039}, {45.015, "Field Reading"=5.46039}, {45.063, "Field Reading"=5.45983}, {45.101, "Field Reading"=5.45983}, {45.157, "Field Reading"=5.45916}, {45.197, "Field Reading"=5.45916}, {45.237, "Field Reading"=5.4586}, {45.289, "Field Reading"=5.4586}, {45.329, "Field Reading"=5.4586}, {45.375, "Field Reading"=5.45798}, {45.414, "Field Reading"=5.45798}, {45.463, "Field Reading"=5.45725}, {45.501, "Field Reading"=5.45725}, {45.557, "Field Reading"=5.45652}, {45.598, "Field Reading"=5.45652}, {45.658, "Field Reading"=5.45557}, {45.696, "Field Reading"=5.45557}, {45.735, "Field Reading"=5.45439}, {45.787, "Field Reading"=5.45439}, {45.827, "Field Reading"=5.45439}, {45.878, "Field Reading"=5.45338}, {45.918, "Field Reading"=5.45338}, {45.977, "Field Reading"=5.45248}, {46.015, "Field Reading"=5.45248}, {46.063, "Field Reading"=5.4517}, {46.101, "Field Reading"=5.4517}, {46.157, "Field Reading"=5.45074}, {46.196, "Field Reading"=5.45074}, {46.235, "Field Reading"=5.45024}, {46.288, "Field Reading"=5.45024}, {46.329, "Field Reading"=5.45024}, {46.375, "Field Reading"=5.44968}, {46.414, "Field Reading"=5.44968}, {46.462, "Field Reading"=5.44895}, {46.501, "Field Reading"=5.44895}, {46.557, "Field Reading"=5.44839}, {46.596, "Field Reading"=5.44839}, {46.636, "Field Reading"=5.44799}, {46.689, "Field Reading"=5.44799}, {46.728, "Field Reading"=5.44799}, {46.776, "Field Reading"=5.44743}, {46.815, "Field Reading"=5.44743}, {46.863, "Field Reading"=5.44682}, {46.902, "Field Reading"=5.44682}, {46.957, "Field Reading"=5.44642}, {46.995, "Field Reading"=5.44642}, {47.034, "Field Reading"=5.44569}, {47.089, "Field Reading"=5.44569}, {47.129, "Field Reading"=5.44569}, {47.176, "Field Reading"=5.44502}, {47.215, "Field Reading"=5.44502}, {47.263, "Field Reading"=5.44446}, {47.302, "Field Reading"=5.44446}, {47.359, "Field Reading"=5.44373}, {47.398, "Field Reading"=5.44373}, {47.438, "Field Reading"=5.44311}, {47.491, "Field Reading"=5.44311}, {47.531, "Field Reading"=5.44311}, {47.577, "Field Reading"=5.4425}, {47.616, "Field Reading"=5.4425}, {47.662, "Field Reading"=5.44177}, {47.703, "Field Reading"=5.44177}, {47.758, "Field Reading"=5.44093}, {47.797, "Field Reading"=5.44093}, {47.837, "Field Reading"=5.4398}, {47.889, "Field Reading"=5.4398}, {47.928, "Field Reading"=5.4398}, {47.976, "Field Reading"=5.43891}, {48.016, "Field Reading"=5.43891}, {48.063, "Field Reading"=5.43801}, {48.102, "Field Reading"=5.43801}, {48.158, "Field Reading"=5.43717}, {48.196, "Field Reading"=5.43717}, {48.233, "Field Reading"=5.43599}, {48.289, "Field Reading"=5.43599}, {48.33, "Field Reading"=5.43599}, {48.376, "Field Reading"=5.43481}, {48.415, "Field Reading"=5.43481}, {48.463, "Field Reading"=5.43363}, {48.502, "Field Reading"=5.43363}, {48.557, "Field Reading"=5.43251}, {48.596, "Field Reading"=5.43251}, {48.634, "Field Reading"=5.43156}, {48.692, "Field Reading"=5.43156}, {48.73, "Field Reading"=5.43156}, {48.777, "Field Reading"=5.43049}, {48.816, "Field Reading"=5.43049}, {48.863, "Field Reading"=5.42954}, {48.901, "Field Reading"=5.42954}, {48.957, "Field Reading"=5.42903}, {48.999, "Field Reading"=5.42903}, {49.058, "Field Reading"=5.42881}, {49.097, "Field Reading"=5.42881}, {49.136, "Field Reading"=5.42881}, {49.19, "Field Reading"=5.42881}, {49.231, "Field Reading"=5.42881}, {49.278, "Field Reading"=5.42881}, {49.317, "Field Reading"=5.42881}, {49.362, "Field Reading"=5.42886}, {49.401, "Field Reading"=5.42886}, {49.459, "Field Reading"=5.42914}, {49.5, "Field Reading"=5.42914}, {49.558, "Field Reading"=5.42931}, {49.596, "Field Reading"=5.42931}, {49.636, "Field Reading"=5.42931}, {49.692, "Field Reading"=5.42931}, {49.731, "Field Reading"=5.42931}, {49.777, "Field Reading"=5.42886}, {49.816, "Field Reading"=5.42886}, {49.864, "Field Reading"=5.42819}, {49.903, "Field Reading"=5.42819}, {49.957, "Field Reading"=5.42741}, {49.996, "Field Reading"=5.42741}, {50.036, "Field Reading"=5.42679}, {50.089, "Field Reading"=5.42679}, {50.13, "Field Reading"=5.42679}, {50.176, "Field Reading"=5.42606}, {50.216, "Field Reading"=5.42606}, {50.264, "Field Reading"=5.42516}, {50.304, "Field Reading"=5.42516}, {50.358, "Field Reading"=5.42443}, {50.397, "Field Reading"=5.42443}, {50.438, "Field Reading"=5.42353}, {50.49, "Field Reading"=5.42353}, {50.53, "Field Reading"=5.42353}, {50.576, "Field Reading"=5.42275}, {50.614, "Field Reading"=5.42275}, {50.664, "Field Reading"=5.42191}, {50.703, "Field Reading"=5.42191}, {50.757, "Field Reading"=5.42101}, {50.798, "Field Reading"=5.42101}, {50.838, "Field Reading"=5.42017}, {50.891, "Field Reading"=5.42017}, {50.93, "Field Reading"=5.42017}, {50.976, "Field Reading"=5.4195}, {51.016, "Field Reading"=5.4195}, {51.063, "Field Reading"=5.4191}, {51.104, "Field Reading"=5.4191}, {51.164, "Field Reading"=5.4186}, {51.204, "Field Reading"=5.4186}, {51.259, "Field Reading"=5.41832}, {51.298, "Field Reading"=5.41832}, {51.336, "Field Reading"=5.41798}, {51.39, "Field Reading"=5.41798}, {51.429, "Field Reading"=5.41798}, {51.478, "Field Reading"=5.4177}, {51.516, "Field Reading"=5.4177}, {51.563, "Field Reading"=5.41714}, {51.601, "Field Reading"=5.41714}, {51.659, "Field Reading"=5.41652}, {51.698, "Field Reading"=5.41652}, {51.737, "Field Reading"=5.41579}, {51.789, "Field Reading"=5.41579}, {51.828, "Field Reading"=5.41579}, {51.878, "Field Reading"=5.41473}, {51.916, "Field Reading"=5.41473}, {51.963, "Field Reading"=5.41349}, {52.004, "Field Reading"=5.41349}, {52.064, "Field Reading"=5.41243}, {52.104, "Field Reading"=5.41243}, {52.159, "Field Reading"=5.41136}, {52.199, "Field Reading"=5.41136}, {52.239, "Field Reading"=5.41018}, {52.292, "Field Reading"=5.41018}, {52.332, "Field Reading"=5.40928}, {52.39, "Field Reading"=5.40928}, {52.43, "Field Reading"=5.40928}, {52.477, "Field Reading"=5.40861}, {52.516, "Field Reading"=5.40861}, {52.563, "Field Reading"=5.40783}, {52.602, "Field Reading"=5.40783}, {52.66, "Field Reading"=5.40732}, {52.699, "Field Reading"=5.40732}, {52.737, "Field Reading"=5.40698}, {52.789, "Field Reading"=5.40698}, {52.827, "Field Reading"=5.40698}, {52.88, "Field Reading"=5.40631}, {52.918, "Field Reading"=5.40631}, {52.963, "Field Reading"=5.40575}, {53.003, "Field Reading"=5.40575}, {53.061, "Field Reading"=5.40513}, {53.101, "Field Reading"=5.40513}, {53.139, "Field Reading"=5.40463}, {53.189, "Field Reading"=5.40463}, {53.231, "Field Reading"=5.40463}, {53.278, "Field Reading"=5.40384}, {53.317, "Field Reading"=5.40384}, {53.363, "Field Reading"=5.40283}, {53.404, "Field Reading"=5.40283}, {53.459, "Field Reading"=5.40177}, {53.499, "Field Reading"=5.40177}, {53.538, "Field Reading"=5.40076}, {53.589, "Field Reading"=5.40076}, {53.628, "Field Reading"=5.40076}, {53.679, "Field Reading"=5.39975}, {53.719, "Field Reading"=5.39975}, {53.765, "Field Reading"=5.39891}, {53.804, "Field Reading"=5.39891}, {53.86, "Field Reading"=5.3979}, {53.9, "Field Reading"=5.3979}, {53.939, "Field Reading"=5.39666}, {53.991, "Field Reading"=5.39666}, {54.029, "Field Reading"=5.39666}, {54.078, "Field Reading"=5.39554}, {54.117, "Field Reading"=5.39554}, {54.164, "Field Reading"=5.39475}, {54.203, "Field Reading"=5.39475}, {54.26, "Field Reading"=5.39386}, {54.299, "Field Reading"=5.39386}, {54.338, "Field Reading"=5.39318}, {54.389, "Field Reading"=5.39318}, {54.43, "Field Reading"=5.39318}, {54.479, "Field Reading"=5.39245}, {54.519, "Field Reading"=5.39245}, {54.564, "Field Reading"=5.39178}, {54.604, "Field Reading"=5.39178}, {54.659, "Field Reading"=5.39139}, {54.698, "Field Reading"=5.39139}, {54.737, "Field Reading"=5.39116}, {54.79, "Field Reading"=5.39116}, {54.831, "Field Reading"=5.39116}, {54.879, "Field Reading"=5.39105}, {54.918, "Field Reading"=5.39105}, {54.964, "Field Reading"=5.39066}, {55.004, "Field Reading"=5.39066}, {55.061, "Field Reading"=5.39027}, {55.1, "Field Reading"=5.39027}, {55.139, "Field Reading"=5.38965}, {55.19, "Field Reading"=5.38965}, {55.23, "Field Reading"=5.38965}, {55.278, "Field Reading"=5.38903}, {55.318, "Field Reading"=5.38903}, {55.364, "Field Reading"=5.3883}, {55.403, "Field Reading"=5.3883}, {55.46, "Field Reading"=5.38763}, {55.499, "Field Reading"=5.38763}, {55.54, "Field Reading"=5.3869}, {55.589, "Field Reading"=5.3869}, {55.63, "Field Reading"=5.3869}, {55.679, "Field Reading"=5.38606}, {55.719, "Field Reading"=5.38606}, {55.764, "Field Reading"=5.38522}, {55.803, "Field Reading"=5.38522}, {55.861, "Field Reading"=5.38426}, {55.9, "Field Reading"=5.38426}, {55.939, "Field Reading"=5.38303}, {55.992, "Field Reading"=5.38303}, {56.031, "Field Reading"=5.38303}, {56.078, "Field Reading"=5.38179}, {56.117, "Field Reading"=5.38179}, {56.165, "Field Reading"=5.38034}, {56.203, "Field Reading"=5.38034}, {56.261, "Field Reading"=5.37899}, {56.301, "Field Reading"=5.37899}, {56.339, "Field Reading"=5.37776}, {56.391, "Field Reading"=5.37776}, {56.433, "Field Reading"=5.3763}, {56.492, "Field Reading"=5.3763}, {56.532, "Field Reading"=5.3763}, {56.579, "Field Reading"=5.37478}, {56.617, "Field Reading"=5.37478}, {56.666, "Field Reading"=5.37346}, {56.705, "Field Reading"=5.37346}, {56.76, "Field Reading"=5.3724}, {56.8, "Field Reading"=5.3724}, {56.84, "Field Reading"=5.37147}, {56.893, "Field Reading"=5.37147}, {56.932, "Field Reading"=5.37147}, {56.98, "Field Reading"=5.37069}, {57.019, "Field Reading"=5.37069}, {57.066, "Field Reading"=5.36965}, {57.106, "Field Reading"=5.36965}, {57.161, "Field Reading"=5.36847}, {57.2, "Field Reading"=5.36847}, {57.238, "Field Reading"=5.36738}, {57.293, "Field Reading"=5.36738}, {57.332, "Field Reading"=5.36738}, {57.379, "Field Reading"=5.36659}, {57.418, "Field Reading"=5.36659}, {57.465, "Field Reading"=5.36589}, {57.505, "Field Reading"=5.36589}, {57.562, "Field Reading"=5.36496}, {57.602, "Field Reading"=5.36496}, {57.661, "Field Reading"=5.36409}, {57.7, "Field Reading"=5.36409}, {57.76, "Field Reading"=5.36328}, {57.799, "Field Reading"=5.36328}, {57.84, "Field Reading"=5.36224}, {57.893, "Field Reading"=5.36224}, {57.931, "Field Reading"=5.36224}, {57.978, "Field Reading"=5.36123}, {58.016, "Field Reading"=5.36123}, {58.067, "Field Reading"=5.36008}, {58.108, "Field Reading"=5.36008}, {58.164, "Field Reading"=5.35877}, {58.205, "Field Reading"=5.35877}, {58.261, "Field Reading"=5.35742}, {58.299, "Field Reading"=5.35742}, {58.338, "Field Reading"=5.35632}, {58.391, "Field Reading"=5.35632}, {58.429, "Field Reading"=5.35632}, {58.479, "Field Reading"=5.35526}, {58.519, "Field Reading"=5.35526}, {58.567, "Field Reading"=5.35447}, {58.605, "Field Reading"=5.35447}, {58.661, "Field Reading"=5.35394}, {58.703, "Field Reading"=5.35394}, {58.76, "Field Reading"=5.35341}, {58.798, "Field Reading"=5.35341}, {58.838, "Field Reading"=5.35324}, {58.892, "Field Reading"=5.35324}, {58.93, "Field Reading"=5.35324}, {58.978, "Field Reading"=5.35307}, {59.017, "Field Reading"=5.35307}, {59.066, "Field Reading"=5.35279}, {59.104, "Field Reading"=5.35279}, {59.16, "Field Reading"=5.35243}, {59.198, "Field Reading"=5.35243}, {59.237, "Field Reading"=5.35189}, {59.292, "Field Reading"=5.35189}, {59.333, "Field Reading"=5.35189}, {59.38, "Field Reading"=5.35111}, {59.418, "Field Reading"=5.35111}, {59.467, "Field Reading"=5.35015}, {59.507, "Field Reading"=5.35015}, {59.562, "Field Reading"=5.34934}, {59.601, "Field Reading"=5.34934}, {59.639, "Field Reading"=5.34844}, {59.693, "Field Reading"=5.34844}, {59.731, "Field Reading"=5.34844}, {59.779, "Field Reading"=5.34749}, {59.817, "Field Reading"=5.34749}, {59.867, "Field Reading"=5.34656}, {59.906, "Field Reading"=5.34656}, {59.961, "Field Reading"=5.34569}, {60.0, "Field Reading"=5.34569}, {60.039, "Field Reading"=5.34474}, {60.093, "Field Reading"=5.34474}, {60.132, "Field Reading"=5.34474}, {60.18, "Field Reading"=5.34376}, {60.219, "Field Reading"=5.34376}, {60.266, "Field Reading"=5.34289}, {60.305, "Field Reading"=5.34289}, {60.36, "Field Reading"=5.34213}, {60.399, "Field Reading"=5.34213}, {60.438, "Field Reading"=5.34123}, {60.494, "Field Reading"=5.34123}, {60.532, "Field Reading"=5.34123}, {60.579, "Field Reading"=5.3405}, {60.617, "Field Reading"=5.3405}, {60.667, "Field Reading"=5.33972}, {60.706, "Field Reading"=5.33972}, {60.761, "Field Reading"=5.33891}, {60.801, "Field Reading"=5.33891}, {60.84, "Field Reading"=5.33823}, {60.892, "Field Reading"=5.33823}, {60.93, "Field Reading"=5.33823}, {60.98, "Field Reading"=5.33773}, {61.019, "Field Reading"=5.33773}, {61.066, "Field Reading"=5.33731}, {61.105, "Field Reading"=5.33731}, {61.16, "Field Reading"=5.33661}, {61.201, "Field Reading"=5.33661}, {61.241, "Field Reading"=5.33604}, {61.292, "Field Reading"=5.33604}, {61.332, "Field Reading"=5.33604}, {61.378, "Field Reading"=5.33537}, {61.417, "Field Reading"=5.33537}, {61.466, "Field Reading"=5.33492}, {61.504, "Field Reading"=5.33492}, {61.56, "Field Reading"=5.33447}, {61.602, "Field Reading"=5.33447}, {61.64, "Field Reading"=5.33374}, {61.693, "Field Reading"=5.33374}, {61.731, "Field Reading"=5.33374}, {61.779, "Field Reading"=5.33287}, {61.82, "Field Reading"=5.33287}, {61.866, "Field Reading"=5.33201}, {61.906, "Field Reading"=5.33201}, {61.966, "Field Reading"=5.3313}, {62.004, "Field Reading"=5.3313}, {62.062, "Field Reading"=5.33055}, {62.101, "Field Reading"=5.33055}, {62.141, "Field Reading"=5.32993}, {62.192, "Field Reading"=5.32993}, {62.231, "Field Reading"=5.32993}, {62.28, "Field Reading"=5.3292}, {62.32, "Field Reading"=5.3292}, {62.366, "Field Reading"=5.32853}, {62.405, "Field Reading"=5.32853}, {62.462, "Field Reading"=5.32785}, {62.501, "Field Reading"=5.32785}, {62.54, "Field Reading"=5.32724}, {62.591, "Field Reading"=5.32724}, {62.633, "Field Reading"=5.32724}, {62.682, "Field Reading"=5.32676}, {62.72, "Field Reading"=5.32676}, {62.766, "Field Reading"=5.32645}, {62.804, "Field Reading"=5.32645}, {62.862, "Field Reading"=5.32614}, {62.9, "Field Reading"=5.32614}, {62.939, "Field Reading"=5.32569}, {62.993, "Field Reading"=5.32569}, {63.035, "Field Reading"=5.32533}, {63.094, "Field Reading"=5.32533}, {63.135, "Field Reading"=5.32533}, {63.181, "Field Reading"=5.32505}, {63.22, "Field Reading"=5.32505}, {63.267, "Field Reading"=5.32494}, {63.308, "Field Reading"=5.32494}, {63.363, "Field Reading"=5.3248}, {63.402, "Field Reading"=5.3248}, {63.462, "Field Reading"=5.3244}, {63.502, "Field Reading"=5.3244}, {63.56, "Field Reading"=5.32404}, {63.6, "Field Reading"=5.32404}, {63.639, "Field Reading"=5.32373}, {63.695, "Field Reading"=5.32373}, {63.734, "Field Reading"=5.32373}, {63.781, "Field Reading"=5.32339}, {63.82, "Field Reading"=5.32339}, {63.867, "Field Reading"=5.32278}, {63.906, "Field Reading"=5.32278}, {63.961, "Field Reading"=5.32202}, {64.0, "Field Reading"=5.32202}, {64.039, "Field Reading"=5.32112}, {64.095, "Field Reading"=5.32112}, {64.133, "Field Reading"=5.32112}, {64.18, "Field Reading"=5.32031}, {64.219, "Field Reading"=5.32031}, {64.267, "Field Reading"=5.31966}, {64.307, "Field Reading"=5.31966}, {64.361, "Field Reading"=5.31874}, {64.402, "Field Reading"=5.31874}, {64.442, "Field Reading"=5.3179}, {64.494, "Field Reading"=5.3179}, {64.533, "Field Reading"=5.3179}, {64.579, "Field Reading"=5.31708}, {64.62, "Field Reading"=5.31708}, {64.669, "Field Reading"=5.3163}, {64.707, "Field Reading"=5.3163}, {64.764, "Field Reading"=5.31565}, {64.804, "Field Reading"=5.31565}, {64.842, "Field Reading"=5.31526}, {64.894, "Field Reading"=5.31526}, {64.934, "Field Reading"=5.31526}, {64.979, "Field Reading"=5.31492}, {65.018, "Field Reading"=5.31492}, {65.068, "Field Reading"=5.31447}, {65.106, "Field Reading"=5.31447}, {65.163, "Field Reading"=5.31431}, {65.203, "Field Reading"=5.31431}, {65.262, "Field Reading"=5.31377}, {65.301, "Field Reading"=5.31377}, {65.339, "Field Reading"=5.31332}, {65.392, "Field Reading"=5.31332}, {65.434, "Field Reading"=5.31332}, {65.481, "Field Reading"=5.31313}, {65.52, "Field Reading"=5.31313}, {65.566, "Field Reading"=5.31276}, {65.606, "Field Reading"=5.31276}, {65.663, "Field Reading"=5.31231}, {65.702, "Field Reading"=5.31231}, {65.741, "Field Reading"=5.31192}, {65.793, "Field Reading"=5.31192}, {65.832, "Field Reading"=5.31192}, {65.881, "Field Reading"=5.31144}, {65.921, "Field Reading"=5.31144}, {65.967, "Field Reading"=5.31111}, {66.006, "Field Reading"=5.31111}, {66.063, "Field Reading"=5.31088}, {66.102, "Field Reading"=5.31088}, {66.141, "Field Reading"=5.31083}, {66.194, "Field Reading"=5.31083}, {66.234, "Field Reading"=5.31083}, {66.282, "Field Reading"=5.3106}, {66.32, "Field Reading"=5.3106}, {66.367, "Field Reading"=5.31046}, {66.406, "Field Reading"=5.31046}, {66.464, "Field Reading"=5.31041}, {66.504, "Field Reading"=5.31041}, {66.543, "Field Reading"=5.31013}, {66.594, "Field Reading"=5.31013}, {66.633, "Field Reading"=5.31013}, {66.681, "Field Reading"=5.30982}, {66.72, "Field Reading"=5.30982}, {66.767, "Field Reading"=5.30928}, {66.805, "Field Reading"=5.30928}, {66.862, "Field Reading"=5.309}, {66.902, "Field Reading"=5.309}, {66.941, "Field Reading"=5.30853}, {66.993, "Field Reading"=5.30853}, {67.034, "Field Reading"=5.30853}, {67.083, "Field Reading"=5.30827}, {67.123, "Field Reading"=5.30827}, {67.167, "Field Reading"=5.30797}, {67.207, "Field Reading"=5.30797}, {67.266, "Field Reading"=5.30749}, {67.305, "Field Reading"=5.30749}, {67.362, "Field Reading"=5.30715}, {67.401, "Field Reading"=5.30715}, {67.442, "Field Reading"=5.3069}, {67.495, "Field Reading"=5.3069}, {67.533, "Field Reading"=5.3069}, {67.581, "Field Reading"=5.30651}, {67.621, "Field Reading"=5.30651}, {67.67, "Field Reading"=5.30609}, {67.711, "Field Reading"=5.30609}, {67.768, "Field Reading"=5.30567}, {67.809, "Field Reading"=5.30567}, {67.865, "Field Reading"=5.30516}, {67.903, "Field Reading"=5.30516}, {67.962, "Field Reading"=5.30466}, {68.0, "Field Reading"=5.30466}, {68.041, "Field Reading"=5.30409}, {68.096, "Field Reading"=5.30409}, {68.135, "Field Reading"=5.30409}, {68.183, "Field Reading"=5.30356}, {68.223, "Field Reading"=5.30356}, {68.269, "Field Reading"=5.30306}, {68.307, "Field Reading"=5.30306}, {68.362, "Field Reading"=5.30261}, {68.402, "Field Reading"=5.30261}, {68.441, "Field Reading"=5.30188}, {68.494, "Field Reading"=5.30188}, {68.534, "Field Reading"=5.30188}, {68.581, "Field Reading"=5.30107}, {68.621, "Field Reading"=5.30107}, {68.668, "Field Reading"=5.30034}, {68.707, "Field Reading"=5.30034}, {68.764, "Field Reading"=5.29952}, {68.803, "Field Reading"=5.29952}, {68.842, "Field Reading"=5.29874}, {68.896, "Field Reading"=5.29874}, {68.935, "Field Reading"=5.29874}, {68.982, "Field Reading"=5.29781}, {69.023, "Field Reading"=5.29781}, {69.068, "Field Reading"=5.29672}, {69.107, "Field Reading"=5.29672}, {69.163, "Field Reading"=5.29551}, {69.203, "Field Reading"=5.29551}, {69.242, "Field Reading"=5.29461}, {69.297, "Field Reading"=5.29461}, {69.335, "Field Reading"=5.29461}, {69.382, "Field Reading"=5.29372}, {69.422, "Field Reading"=5.29372}, {69.469, "Field Reading"=5.29282}, {69.509, "Field Reading"=5.29282}, {69.565, "Field Reading"=5.29209}, {69.605, "Field Reading"=5.29209}, {69.664, "Field Reading"=5.29116}, {69.703, "Field Reading"=5.29116}, {69.742, "Field Reading"=5.29035}, {69.797, "Field Reading"=5.29035}, {69.838, "Field Reading"=5.2899}, {69.895, "Field Reading"=5.2899}, {69.934, "Field Reading"=5.2899}, {69.982, "Field Reading"=5.28956}, {70.02, "Field Reading"=5.28956}, {70.069, "Field Reading"=5.28923}, {70.109, "Field Reading"=5.28923}, {70.165, "Field Reading"=5.28892}, {70.204, "Field Reading"=5.28892}, {70.243, "Field Reading"=5.2885}, {70.296, "Field Reading"=5.2885}, {70.336, "Field Reading"=5.2885}, {70.383, "Field Reading"=5.2878}, {70.422, "Field Reading"=5.2878}, {70.469, "Field Reading"=5.28746}, {70.509, "Field Reading"=5.28746}, {70.565, "Field Reading"=5.2871}, {70.605, "Field Reading"=5.2871}, {70.664, "Field Reading"=5.28634}, {70.705, "Field Reading"=5.28634}, {70.764, "Field Reading"=5.28564}, {70.802, "Field Reading"=5.28564}, {70.843, "Field Reading"=5.2851}, {70.896, "Field Reading"=5.2851}, {70.934, "Field Reading"=5.2851}, {70.982, "Field Reading"=5.28454}, {71.021, "Field Reading"=5.28454}, {71.071, "Field Reading"=5.28401}, {71.112, "Field Reading"=5.28401}, {71.17, "Field Reading"=5.28367}, {71.21, "Field Reading"=5.28367}, {71.27, "Field Reading"=5.28317}, {71.31, "Field Reading"=5.28317}, {71.369, "Field Reading"=5.28286}, {71.408, "Field Reading"=5.28286}, {71.464, "Field Reading"=5.2828}, {71.503, "Field Reading"=5.2828}, {71.543, "Field Reading"=5.28266}, {71.595, "Field Reading"=5.28266}, {71.634, "Field Reading"=5.28266}, {71.684, "Field Reading"=5.28244}, {71.723, "Field Reading"=5.28244}, {71.77, "Field Reading"=5.2821}, {71.81, "Field Reading"=5.2821}, {71.869, "Field Reading"=5.28185}, {71.909, "Field Reading"=5.28185}, {71.964, "Field Reading"=5.28143}, {72.004, "Field Reading"=5.28143}, {72.065, "Field Reading"=5.28126}, {72.103, "Field Reading"=5.28126}, {72.142, "Field Reading"=5.28079}, {72.195, "Field Reading"=5.28079}, {72.234, "Field Reading"=5.28079}, {72.284, "Field Reading"=5.28036}, {72.323, "Field Reading"=5.28036}, {72.369, "Field Reading"=5.27986}, {72.41, "Field Reading"=5.27986}, {72.467, "Field Reading"=5.27905}, {72.506, "Field Reading"=5.27905}, {72.564, "Field Reading"=5.27829}, {72.602, "Field Reading"=5.27829}, {72.642, "Field Reading"=5.27745}, {72.695, "Field Reading"=5.27745}, {72.734, "Field Reading"=5.27745}, {72.783, "Field Reading"=5.2768}, {72.824, "Field Reading"=5.2768}, {72.869, "Field Reading"=5.27596}, {72.909, "Field Reading"=5.27596}, {72.964, "Field Reading"=5.27515}, {73.004, "Field Reading"=5.27515}, {73.044, "Field Reading"=5.27422}, {73.098, "Field Reading"=5.27422}, {73.137, "Field Reading"=5.27422}, {73.184, "Field Reading"=5.27346}, {73.224, "Field Reading"=5.27346}, {73.27, "Field Reading"=5.27296}, {73.309, "Field Reading"=5.27296}, {73.365, "Field Reading"=5.27251}, {73.405, "Field Reading"=5.27251}, {73.444, "Field Reading"=5.27209}, {73.497, "Field Reading"=5.27209}, {73.536, "Field Reading"=5.27209}, {73.583, "Field Reading"=5.2715}, {73.625, "Field Reading"=5.2715}, {73.685, "Field Reading"=5.27091}, {73.724, "Field Reading"=5.27091}, {73.769, "Field Reading"=5.27057}, {73.809, "Field Reading"=5.27057}, {73.865, "Field Reading"=5.27024}, {73.906, "Field Reading"=5.27024}, {73.964, "Field Reading"=5.27007}, {74.004, "Field Reading"=5.27007}, {74.044, "Field Reading"=5.26987}, {74.097, "Field Reading"=5.26987}, {74.137, "Field Reading"=5.26987}, {74.185, "Field Reading"=5.26976}, {74.226, "Field Reading"=5.26976}, {74.284, "Field Reading"=5.2699}, {74.323, "Field Reading"=5.2699}, {74.369, "Field Reading"=5.27004}, {74.411, "Field Reading"=5.27004}, {74.47, "Field Reading"=5.27038}, {74.508, "Field Reading"=5.27038}, {74.564, "Field Reading"=5.27057}, {74.604, "Field Reading"=5.27057}, {74.665, "Field Reading"=5.27063}, {74.704, "Field Reading"=5.27063}, {74.764, "Field Reading"=5.27057}, {74.803, "Field Reading"=5.27057}, {74.843, "Field Reading"=5.27046}, {74.899, "Field Reading"=5.27046}, {74.937, "Field Reading"=5.27046}, {74.985, "Field Reading"=5.27029}, {75.027, "Field Reading"=5.27029}, {75.083, "Field Reading"=5.27007}, {75.122, "Field Reading"=5.27007}, {75.17, "Field Reading"=5.2701}, {75.211, "Field Reading"=5.2701}, {75.268, "Field Reading"=5.27004}, {75.309, "Field Reading"=5.27004}, {75.367, "Field Reading"=5.26996}, {75.406, "Field Reading"=5.26996}, {75.465, "Field Reading"=5.26996}, {75.504, "Field Reading"=5.26996}, {75.565, "Field Reading"=5.27004}, {75.606, "Field Reading"=5.27004}, {75.666, "Field Reading"=5.27027}, {75.707, "Field Reading"=5.27027}, {75.764, "Field Reading"=5.27038}, {75.803, "Field Reading"=5.27038}, {75.842, "Field Reading"=5.2706}, {75.899, "Field Reading"=5.2706}, {75.939, "Field Reading"=5.27077}, {75.995, "Field Reading"=5.27077}, {76.035, "Field Reading"=5.27077}, {76.085, "Field Reading"=5.27128}, {76.125, "Field Reading"=5.27128}, {76.184, "Field Reading"=5.27161}, {76.223, "Field Reading"=5.27161}, {76.27, "Field Reading"=5.27206}, {76.309, "Field Reading"=5.27206}, {76.364, "Field Reading"=5.27248}, {76.403, "Field Reading"=5.27248}, {76.444, "Field Reading"=5.27296}, {76.496, "Field Reading"=5.27296}, {76.536, "Field Reading"=5.27296}, {76.585, "Field Reading"=5.27332}, {76.624, "Field Reading"=5.27332}, {76.671, "Field Reading"=5.27363}, {76.711, "Field Reading"=5.27363}, {76.769, "Field Reading"=5.27383}, {76.808, "Field Reading"=5.27383}, {76.866, "Field Reading"=5.27374}, {76.905, "Field Reading"=5.27374}, {76.945, "Field Reading"=5.2738}, {76.997, "Field Reading"=5.2738}, {77.036, "Field Reading"=5.2738}, {77.085, "Field Reading"=5.27374}, {77.123, "Field Reading"=5.27374}, {77.17, "Field Reading"=5.27352}, {77.21, "Field Reading"=5.27352}, {77.268, "Field Reading"=5.27321}, {77.308, "Field Reading"=5.27321}, {77.365, "Field Reading"=5.27324}, {77.404, "Field Reading"=5.27324}, {77.442, "Field Reading"=5.27313}, {77.5, "Field Reading"=5.27313}, {77.54, "Field Reading"=5.27302}, {77.597, "Field Reading"=5.27302}, {77.636, "Field Reading"=5.27302}, {77.684, "Field Reading"=5.27307}, {77.723, "Field Reading"=5.27307}, {77.77, "Field Reading"=5.27302}, {77.809, "Field Reading"=5.27302}, {77.866, "Field Reading"=5.27304}, {77.905, "Field Reading"=5.27304}, {77.945, "Field Reading"=5.27318}, {77.996, "Field Reading"=5.27318}, {78.036, "Field Reading"=5.27318}, {78.085, "Field Reading"=5.27327}, {78.125, "Field Reading"=5.27327}, {78.17, "Field Reading"=5.27324}, {78.211, "Field Reading"=5.27324}, {78.268, "Field Reading"=5.27327}, {78.308, "Field Reading"=5.27327}, {78.365, "Field Reading"=5.2731}, {78.406, "Field Reading"=5.2731}, {78.445, "Field Reading"=5.27262}, {78.497, "Field Reading"=5.27262}, {78.538, "Field Reading"=5.27262}, {78.586, "Field Reading"=5.27231}, {78.626, "Field Reading"=5.27231}, {78.685, "Field Reading"=5.27198}, {78.726, "Field Reading"=5.27198}, {78.771, "Field Reading"=5.27158}, {78.809, "Field Reading"=5.27158}, {78.867, "Field Reading"=5.27114}, {78.907, "Field Reading"=5.27114}, {78.946, "Field Reading"=5.27074}, {78.999, "Field Reading"=5.27074}, {79.038, "Field Reading"=5.27074}, {79.087, "Field Reading"=5.27038}, {79.126, "Field Reading"=5.27038}, {79.17, "Field Reading"=5.27013}, {79.21, "Field Reading"=5.27013}, {79.268, "Field Reading"=5.27018}, {79.309, "Field Reading"=5.27018}, {79.366, "Field Reading"=5.27007}, {79.406, "Field Reading"=5.27007}, {79.445, "Field Reading"=5.26999}, {79.497, "Field Reading"=5.26999}, {79.539, "Field Reading"=5.26976}, {79.596, "Field Reading"=5.26976}, {79.636, "Field Reading"=5.26976}, {79.687, "Field Reading"=5.26968}, {79.727, "Field Reading"=5.26968}, {79.784, "Field Reading"=5.26928}, {79.824, "Field Reading"=5.26928}, {79.874, "Field Reading"=5.26878}, {79.914, "Field Reading"=5.26878}, {79.97, "Field Reading"=5.26839}, {80.011, "Field Reading"=5.26839}, {80.067, "Field Reading"=5.26791}, {80.106, "Field Reading"=5.26791}, {80.145, "Field Reading"=5.26732}, {80.197, "Field Reading"=5.26732}, {80.236, "Field Reading"=5.26732}, {80.286, "Field Reading"=5.26679}, {80.325, "Field Reading"=5.26679}, {80.372, "Field Reading"=5.2664}, {80.411, "Field Reading"=5.2664}, {80.472, "Field Reading"=5.26589}, {80.511, "Field Reading"=5.26589}, {80.567, "Field Reading"=5.26553}, {80.605, "Field Reading"=5.26553}, {80.644, "Field Reading"=5.26513}, {80.699, "Field Reading"=5.26513}, {80.739, "Field Reading"=5.26468}, {80.796, "Field Reading"=5.26468}, {80.837, "Field Reading"=5.26468}, {80.886, "Field Reading"=5.26415}, {80.926, "Field Reading"=5.26415}, {80.971, "Field Reading"=5.26337}, {81.01, "Field Reading"=5.26337}, {81.067, "Field Reading"=5.26241}, {81.106, "Field Reading"=5.26241}, {81.145, "Field Reading"=5.26132}, {81.2, "Field Reading"=5.26132}, {81.239, "Field Reading"=5.26132}, {81.286, "Field Reading"=5.26006}, {81.325, "Field Reading"=5.26006}, {81.371, "Field Reading"=5.25891}, {81.41, "Field Reading"=5.25891}, {81.467, "Field Reading"=5.25764}, {81.506, "Field Reading"=5.25764}, {81.545, "Field Reading"=5.25641}, {81.597, "Field Reading"=5.25641}, {81.637, "Field Reading"=5.25641}, {81.686, "Field Reading"=5.25523}, {81.725, "Field Reading"=5.25523}, {81.773, "Field Reading"=5.25433}, {81.812, "Field Reading"=5.25433}, {81.869, "Field Reading"=5.25358}, {81.911, "Field Reading"=5.25358}, {81.966, "Field Reading"=5.25307}, {82.007, "Field Reading"=5.25307}, {82.046, "Field Reading"=5.25265}, {82.1, "Field Reading"=5.25265}, {82.14, "Field Reading"=5.25209}, {82.199, "Field Reading"=5.25209}, {82.238, "Field Reading"=5.25209}, {82.287, "Field Reading"=5.25161}, {82.325, "Field Reading"=5.25161}, {82.372, "Field Reading"=5.251}, {82.413, "Field Reading"=5.251}, {82.473, "Field Reading"=5.25035}, {82.514, "Field Reading"=5.25035}, {82.571, "Field Reading"=5.24968}, {82.61, "Field Reading"=5.24968}, {82.668, "Field Reading"=5.24872}, {82.707, "Field Reading"=5.24872}, {82.746, "Field Reading"=5.24816}, {82.798, "Field Reading"=5.24816}, {82.838, "Field Reading"=5.24816}, {82.886, "Field Reading"=5.24755}, {82.925, "Field Reading"=5.24755}, {82.973, "Field Reading"=5.24696}, {83.013, "Field Reading"=5.24696}, {83.072, "Field Reading"=5.24628}, {83.111, "Field Reading"=5.24628}, {83.168, "Field Reading"=5.24567}, {83.208, "Field Reading"=5.24567}, {83.267, "Field Reading"=5.24499}, {83.308, "Field Reading"=5.24499}, {83.366, "Field Reading"=5.24429}, {83.405, "Field Reading"=5.24429}, {83.445, "Field Reading"=5.24376}, {83.499, "Field Reading"=5.24376}, {83.539, "Field Reading"=5.24376}, {83.586, "Field Reading"=5.24286}, {83.627, "Field Reading"=5.24286}, {83.672, "Field Reading"=5.24224}, {83.712, "Field Reading"=5.24224}, {83.768, "Field Reading"=5.24132}, {83.807, "Field Reading"=5.24132}, {83.868, "Field Reading"=5.24073}, {83.907, "Field Reading"=5.24073}, {83.946, "Field Reading"=5.24017}, {83.999, "Field Reading"=5.24017}, {84.039, "Field Reading"=5.24017}, {84.087, "Field Reading"=5.23961}, {84.127, "Field Reading"=5.23961}, {84.172, "Field Reading"=5.23905}, {84.211, "Field Reading"=5.23905}, {84.267, "Field Reading"=5.23851}, {84.307, "Field Reading"=5.23851}, {84.347, "Field Reading"=5.23792}, {84.398, "Field Reading"=5.23792}, {84.437, "Field Reading"=5.23792}, {84.489, "Field Reading"=5.23708}, {84.528, "Field Reading"=5.23708}, {84.573, "Field Reading"=5.23663}, {84.613, "Field Reading"=5.23663}, {84.669, "Field Reading"=5.23596}, {84.708, "Field Reading"=5.23596}, {84.767, "Field Reading"=5.23532}, {84.807, "Field Reading"=5.23532}, {84.846, "Field Reading"=5.2347}, {84.899, "Field Reading"=5.2347}, {84.938, "Field Reading"=5.2347}, {84.986, "Field Reading"=5.23428}, {85.026, "Field Reading"=5.23428}, {85.073, "Field Reading"=5.23408}, {85.114, "Field Reading"=5.23408}, {85.172, "Field Reading"=5.23386}, {85.213, "Field Reading"=5.23386}, {85.272, "Field Reading"=5.23369}, {85.313, "Field Reading"=5.23369}, {85.368, "Field Reading"=5.23349}, {85.406, "Field Reading"=5.23349}, {85.446, "Field Reading"=5.23349}, {85.499, "Field Reading"=5.23349}, {85.539, "Field Reading"=5.23349}, {85.586, "Field Reading"=5.23358}, {85.627, "Field Reading"=5.23358}, {85.673, "Field Reading"=5.23369}, {85.713, "Field Reading"=5.23369}, {85.768, "Field Reading"=5.23369}, {85.809, "Field Reading"=5.23369}, {85.848, "Field Reading"=5.23341}, {85.899, "Field Reading"=5.23341}, {85.938, "Field Reading"=5.23341}, {85.986, "Field Reading"=5.23316}, {86.024, "Field Reading"=5.23316}, {86.073, "Field Reading"=5.23273}, {86.112, "Field Reading"=5.23273}, {86.169, "Field Reading"=5.23229}, {86.208, "Field Reading"=5.23229}, {86.247, "Field Reading"=5.2315}, {86.301, "Field Reading"=5.2315}, {86.341, "Field Reading"=5.23063}, {86.399, "Field Reading"=5.23063}, {86.437, "Field Reading"=5.23063}, {86.488, "Field Reading"=5.22993}, {86.527, "Field Reading"=5.22993}, {86.572, "Field Reading"=5.22959}, {86.614, "Field Reading"=5.22959}, {86.673, "Field Reading"=5.22937}, {86.714, "Field Reading"=5.22937}, {86.77, "Field Reading"=5.22928}, {86.809, "Field Reading"=5.22928}, {86.848, "Field Reading"=5.22951}, {86.902, "Field Reading"=5.22951}, {86.942, "Field Reading"=5.22976}, {86.998, "Field Reading"=5.22976}, {87.039, "Field Reading"=5.22976}, {87.088, "Field Reading"=5.23021}, {87.128, "Field Reading"=5.23021}, {87.173, "Field Reading"=5.23052}, {87.211, "Field Reading"=5.23052}, {87.268, "Field Reading"=5.23088}, {87.308, "Field Reading"=5.23088}, {87.347, "Field Reading"=5.231}, {87.399, "Field Reading"=5.231}, {87.44, "Field Reading"=5.231}, {87.489, "Field Reading"=5.23125}, {87.527, "Field Reading"=5.23125}, {87.573, "Field Reading"=5.23142}, {87.612, "Field Reading"=5.23142}, {87.67, "Field Reading"=5.2315}, {87.709, "Field Reading"=5.2315}, {87.749, "Field Reading"=5.23147}, {87.8, "Field Reading"=5.23147}, {87.839, "Field Reading"=5.23147}, {87.887, "Field Reading"=5.23158}, {87.929, "Field Reading"=5.23158}, {87.986, "Field Reading"=5.23203}, {88.025, "Field Reading"=5.23203}, {88.074, "Field Reading"=5.23231}, {88.114, "Field Reading"=5.23231}, {88.169, "Field Reading"=5.23273}, {88.208, "Field Reading"=5.23273}, {88.247, "Field Reading"=5.23307}, {88.299, "Field Reading"=5.23307}, {88.338, "Field Reading"=5.23307}, {88.387, "Field Reading"=5.23335}, {88.426, "Field Reading"=5.23335}, {88.474, "Field Reading"=5.23358}, {88.512, "Field Reading"=5.23358}, {88.567, "Field Reading"=5.23383}, {88.609, "Field Reading"=5.23383}, {88.648, "Field Reading"=5.23402}, {88.703, "Field Reading"=5.23402}, {88.742, "Field Reading"=5.23422}, {88.801, "Field Reading"=5.23422}, {88.839, "Field Reading"=5.23422}, {88.89, "Field Reading"=5.23439}, {88.93, "Field Reading"=5.23439}, {88.989, "Field Reading"=5.23433}, {89.027, "Field Reading"=5.23433}, {89.076, "Field Reading"=5.23402}, {89.117, "Field Reading"=5.23402}, {89.175, "Field Reading"=5.23369}, {89.214, "Field Reading"=5.23369}, {89.274, "Field Reading"=5.23327}, {89.311, "Field Reading"=5.23327}, {89.37, "Field Reading"=5.23302}, {89.408, "Field Reading"=5.23302}, {89.447, "Field Reading"=5.23265}, {89.502, "Field Reading"=5.23265}, {89.543, "Field Reading"=5.2322}, {89.602, "Field Reading"=5.2322}, {89.642, "Field Reading"=5.23175}, {89.702, "Field Reading"=5.23175}, {89.742, "Field Reading"=5.23108}, {89.801, "Field Reading"=5.23108}, {89.84, "Field Reading"=5.23108}, {89.89, "Field Reading"=5.2306}, {89.929, "Field Reading"=5.2306}, {89.989, "Field Reading"=5.23018}, {90.027, "Field Reading"=5.23018}, {90.076, "Field Reading"=5.2299}, {90.117, "Field Reading"=5.2299}, {90.175, "Field Reading"=5.22979}, {90.214, "Field Reading"=5.22979}, {90.274, "Field Reading"=5.22976}, {90.313, "Field Reading"=5.22976}, {90.37, "Field Reading"=5.22968}, {90.409, "Field Reading"=5.22968}, {90.448, "Field Reading"=5.22951}, {90.504, "Field Reading"=5.22951}, {90.543, "Field Reading"=5.22962}, {90.601, "Field Reading"=5.22962}, {90.639, "Field Reading"=5.22962}, {90.69, "Field Reading"=5.22962}, {90.73, "Field Reading"=5.22962}, {90.789, "Field Reading"=5.22976}, {90.829, "Field Reading"=5.22976}, {90.878, "Field Reading"=5.22968}, {90.918, "Field Reading"=5.22968}, {90.976, "Field Reading"=5.22923}, {91.016, "Field Reading"=5.22923}, {91.074, "Field Reading"=5.22886}, {91.112, "Field Reading"=5.22886}, {91.17, "Field Reading"=5.22847}, {91.208, "Field Reading"=5.22847}, {91.247, "Field Reading"=5.22822}, {91.305, "Field Reading"=5.22822}, {91.344, "Field Reading"=5.22799}, {91.403, "Field Reading"=5.22799}, {91.443, "Field Reading"=5.22791}, {91.503, "Field Reading"=5.22791}, {91.543, "Field Reading"=5.2276}, {91.602, "Field Reading"=5.2276}, {91.642, "Field Reading"=5.2276}, {91.692, "Field Reading"=5.22755}, {91.731, "Field Reading"=5.22755}, {91.789, "Field Reading"=5.22749}, {91.827, "Field Reading"=5.22749}, {91.877, "Field Reading"=5.22746}, {91.916, "Field Reading"=5.22746}, {91.976, "Field Reading"=5.22729}, {92.015, "Field Reading"=5.22729}, {92.074, "Field Reading"=5.22696}, {92.114, "Field Reading"=5.22696}, {92.176, "Field Reading"=5.22645}, {92.217, "Field Reading"=5.22645}, {92.276, "Field Reading"=5.22589}, {92.316, "Field Reading"=5.22589}, {92.376, "Field Reading"=5.22536}, {92.417, "Field Reading"=5.22536}, {92.477, "Field Reading"=5.22471}, {92.515, "Field Reading"=5.22471}, {92.572, "Field Reading"=5.22393}, {92.611, "Field Reading"=5.22393}, {92.672, "Field Reading"=5.22323}, {92.711, "Field Reading"=5.22323}, {92.771, "Field Reading"=5.22264}, {92.809, "Field Reading"=5.22264}, {92.872, "Field Reading"=5.22241}, {92.91, "Field Reading"=5.22241}, {92.949, "Field Reading"=5.2221}, {93.002, "Field Reading"=5.2221}, {93.042, "Field Reading"=5.22185}, {93.104, "Field Reading"=5.22185}, {93.143, "Field Reading"=5.22174}, {93.202, "Field Reading"=5.22174}, {93.241, "Field Reading"=5.22174}, {93.291, "Field Reading"=5.22174}, {93.332, "Field Reading"=5.22174}, {93.39, "Field Reading"=5.22191}, {93.429, "Field Reading"=5.22191}, {93.477, "Field Reading"=5.22191}, {93.517, "Field Reading"=5.22191}, {93.574, "Field Reading"=5.22171}, {93.613, "Field Reading"=5.22171}, {93.672, "Field Reading"=5.22129}, {93.711, "Field Reading"=5.22129}, {93.75, "Field Reading"=5.2209}, {93.804, "Field Reading"=5.2209}, {93.844, "Field Reading"=5.22045}, {93.903, "Field Reading"=5.22045}, {93.944, "Field Reading"=5.21974}, {94.004, "Field Reading"=5.21974}, {94.044, "Field Reading"=5.21906}, {94.104, "Field Reading"=5.21906}, {94.143, "Field Reading"=5.21848}, {94.202, "Field Reading"=5.21848}, {94.242, "Field Reading"=5.21848}, {94.292, "Field Reading"=5.21785}, {94.332, "Field Reading"=5.21785}, {94.39, "Field Reading"=5.21717}, {94.429, "Field Reading"=5.21717}, {94.478, "Field Reading"=5.21633}, {94.517, "Field Reading"=5.21633}, {94.576, "Field Reading"=5.21576}, {94.617, "Field Reading"=5.21576}, {94.678, "Field Reading"=5.21539}, {94.718, "Field Reading"=5.21539}, {94.776, "Field Reading"=5.21507}, {94.817, "Field Reading"=5.21507}, {94.877, "Field Reading"=5.2146}, {94.916, "Field Reading"=5.2146}, {94.973, "Field Reading"=5.21397}, {95.012, "Field Reading"=5.21397}, {95.072, "Field Reading"=5.2134}, {95.112, "Field Reading"=5.2134}, {95.171, "Field Reading"=5.21277}, {95.21, "Field Reading"=5.21277}, {95.248, "Field Reading"=5.2124}, {95.305, "Field Reading"=5.2124}, {95.344, "Field Reading"=5.21183}, {95.404, "Field Reading"=5.21183}, {95.442, "Field Reading"=5.21183}, {95.492, "Field Reading"=5.2113}, {95.531, "Field Reading"=5.2113}, {95.59, "Field Reading"=5.21083}, {95.628, "Field Reading"=5.21083}, {95.677, "Field Reading"=5.21057}, {95.718, "Field Reading"=5.21057}, {95.776, "Field Reading"=5.21025}, {95.816, "Field Reading"=5.21025}, {95.878, "Field Reading"=5.20983}, {95.919, "Field Reading"=5.20983}, {95.976, "Field Reading"=5.20968}, {96.016, "Field Reading"=5.20968}, {96.076, "Field Reading"=5.20942}, {96.117, "Field Reading"=5.20942}, {96.174, "Field Reading"=5.20915}, {96.214, "Field Reading"=5.20915}, {96.273, "Field Reading"=5.20858}, {96.311, "Field Reading"=5.20858}, {96.35, "Field Reading"=5.2079}, {96.402, "Field Reading"=5.2079}, {96.441, "Field Reading"=5.2079}, {96.491, "Field Reading"=5.20711}, {96.531, "Field Reading"=5.20711}, {96.59, "Field Reading"=5.20632}, {96.629, "Field Reading"=5.20632}, {96.679, "Field Reading"=5.2058}, {96.718, "Field Reading"=5.2058}, {96.777, "Field Reading"=5.20522}, {96.816, "Field Reading"=5.20522}, {96.874, "Field Reading"=5.20454}, {96.914, "Field Reading"=5.20454}, {96.972, "Field Reading"=5.20391}, {97.013, "Field Reading"=5.20391}, {97.073, "Field Reading"=5.20328}, {97.113, "Field Reading"=5.20328}, {97.172, "Field Reading"=5.20271}, {97.211, "Field Reading"=5.20271}, {97.249, "Field Reading"=5.20197}, {97.305, "Field Reading"=5.20197}, {97.345, "Field Reading"=5.20129}, {97.402, "Field Reading"=5.20129}, {97.443, "Field Reading"=5.20129}, {97.492, "Field Reading"=5.20066}, {97.533, "Field Reading"=5.20066}, {97.59, "Field Reading"=5.19993}, {97.628, "Field Reading"=5.19993}, {97.678, "Field Reading"=5.19914}, {97.717, "Field Reading"=5.19914}, {97.774, "Field Reading"=5.19846}, {97.813, "Field Reading"=5.19846}, {97.873, "Field Reading"=5.19783}, {97.912, "Field Reading"=5.19783}, {97.95, "Field Reading"=5.19731}, {98.004, "Field Reading"=5.19731}, {98.043, "Field Reading"=5.19731}, {98.092, "Field Reading"=5.19684}, {98.13, "Field Reading"=5.19684}, {98.178, "Field Reading"=5.19647}, {98.217, "Field Reading"=5.19647}, {98.278, "Field Reading"=5.19595}, {98.317, "Field Reading"=5.19595}, {98.374, "Field Reading"=5.19527}, {98.412, "Field Reading"=5.19527}, {98.473, "Field Reading"=5.19469}, {98.513, "Field Reading"=5.19469}, {98.572, "Field Reading"=5.19411}, {98.61, "Field Reading"=5.19411}, {98.651, "Field Reading"=5.19349}, {98.706, "Field Reading"=5.19349}, {98.746, "Field Reading"=5.19291}, {98.805, "Field Reading"=5.19291}, {98.847, "Field Reading"=5.19228}, {98.905, "Field Reading"=5.19228}, {98.944, "Field Reading"=5.19155}, {99.003, "Field Reading"=5.19155}, {99.044, "Field Reading"=5.19081}, {99.106, "Field Reading"=5.19081}, {99.145, "Field Reading"=5.19039}, {99.205, "Field Reading"=5.19039}, {99.242, "Field Reading"=5.19039}, {99.293, "Field Reading"=5.19003}, {99.332, "Field Reading"=5.19003}, {99.392, "Field Reading"=5.18956}, {99.431, "Field Reading"=5.18956}, {99.48, "Field Reading"=5.18908}, {99.519, "Field Reading"=5.18908}, {99.579, "Field Reading"=5.18861}, {99.617, "Field Reading"=5.18861}, {99.675, "Field Reading"=5.18814}, {99.715, "Field Reading"=5.18814}, {99.772, "Field Reading"=5.18767}, {99.812, "Field Reading"=5.18767}, {99.85, "Field Reading"=5.18709}, {99.905, "Field Reading"=5.18709}, {99.945, "Field Reading"=5.18657}, {100.004, "Field Reading"=5.18657}, {100.044, "Field Reading"=5.18589}, {100.106, "Field Reading"=5.18589}, {100.145, "Field Reading"=5.18526}, {100.203, "Field Reading"=5.18526}, {100.241, "Field Reading"=5.18526}, {100.292, "Field Reading"=5.18463}, {100.331, "Field Reading"=5.18463}, {100.378, "Field Reading"=5.184}, {100.417, "Field Reading"=5.184}, {100.475, "Field Reading"=5.18316}, {100.516, "Field Reading"=5.18316}, {100.574, "Field Reading"=5.18238}, {100.613, "Field Reading"=5.18238}, {100.651, "Field Reading"=5.18159}, {100.705, "Field Reading"=5.18159}, {100.745, "Field Reading"=5.18054}, {100.805, "Field Reading"=5.18054}, {100.845, "Field Reading"=5.17955}, {100.906, "Field Reading"=5.17955}, {100.946, "Field Reading"=5.17855}, {101.004, "Field Reading"=5.17855}, {101.043, "Field Reading"=5.17855}, {101.093, "Field Reading"=5.17766}, {101.131, "Field Reading"=5.17766}, {101.178, "Field Reading"=5.17682}, {101.217, "Field Reading"=5.17682}, {101.275, "Field Reading"=5.17603}, {101.313, "Field Reading"=5.17603}, {101.351, "Field Reading"=5.17535}, {101.406, "Field Reading"=5.17535}, {101.447, "Field Reading"=5.17483}, {101.505, "Field Reading"=5.17483}, {101.543, "Field Reading"=5.17483}, {101.593, "Field Reading"=5.17425}, {101.633, "Field Reading"=5.17425}, {101.693, "Field Reading"=5.17357}, {101.734, "Field Reading"=5.17357}, {101.791, "Field Reading"=5.17289}, {101.83, "Field Reading"=5.17289}, {101.879, "Field Reading"=5.172}, {101.917, "Field Reading"=5.172}, {101.975, "Field Reading"=5.17106}, {102.015, "Field Reading"=5.17106}, {102.074, "Field Reading"=5.17022}, {102.113, "Field Reading"=5.17022}, {102.174, "Field Reading"=5.16938}, {102.211, "Field Reading"=5.16938}, {102.25, "Field Reading"=5.16833}, {102.306, "Field Reading"=5.16833}, {102.345, "Field Reading"=5.16833}, {102.395, "Field Reading"=5.16739}, {102.436, "Field Reading"=5.16739}, {102.493, "Field Reading"=5.16645}, {102.531, "Field Reading"=5.16645}, {102.579, "Field Reading"=5.1655}, {102.617, "Field Reading"=5.1655}, {102.677, "Field Reading"=5.16445}, {102.715, "Field Reading"=5.16445}, {102.774, "Field Reading"=5.16356}, {102.813, "Field Reading"=5.16356}, {102.875, "Field Reading"=5.16273}, {102.914, "Field Reading"=5.16273}, {102.974, "Field Reading"=5.16178}, {103.011, "Field Reading"=5.16178}, {103.05, "Field Reading"=5.1611}, {103.105, "Field Reading"=5.1611}, {103.145, "Field Reading"=5.16042}, {103.206, "Field Reading"=5.16042}, {103.246, "Field Reading"=5.16016}, {103.307, "Field Reading"=5.16016}, {103.347, "Field Reading"=5.15979}, {103.406, "Field Reading"=5.15979}, {103.447, "Field Reading"=5.15969}, {103.507, "Field Reading"=5.15969}, {103.546, "Field Reading"=5.15969}, {103.605, "Field Reading"=5.15969}, {103.645, "Field Reading"=5.15979}, {103.706, "Field Reading"=5.15979}, {103.746, "Field Reading"=5.15984}, {103.804, "Field Reading"=5.15984}, {103.845, "Field Reading"=5.15984}, {103.894, "Field Reading"=5.15984}, {103.932, "Field Reading"=5.15984}, {103.979, "Field Reading"=5.15974}, {104.019, "Field Reading"=5.15974}, {104.077, "Field Reading"=5.15932}, {104.117, "Field Reading"=5.15932}, {104.175, "Field Reading"=5.1588}, {104.214, "Field Reading"=5.1588}, {104.275, "Field Reading"=5.15827}, {104.314, "Field Reading"=5.15827}, {104.374, "Field Reading"=5.15769}, {104.413, "Field Reading"=5.15769}, {104.453, "Field Reading"=5.15686}, {104.506, "Field Reading"=5.15686}, {104.547, "Field Reading"=5.15607}, {104.605, "Field Reading"=5.15607}, {104.645, "Field Reading"=5.15539}, {104.707, "Field Reading"=5.15539}, {104.748, "Field Reading"=5.15476}, {104.805, "Field Reading"=5.15476}, {104.847, "Field Reading"=5.15418}, {104.908, "Field Reading"=5.15418}, {104.947, "Field Reading"=5.15376}, {105.007, "Field Reading"=5.15376}, {105.046, "Field Reading"=5.15324}, {105.105, "Field Reading"=5.15324}, {105.144, "Field Reading"=5.15324}, {105.192, "Field Reading"=5.15266}, {105.23, "Field Reading"=5.15266}, {105.28, "Field Reading"=5.15219}, {105.321, "Field Reading"=5.15219}, {105.379, "Field Reading"=5.15193}, {105.42, "Field Reading"=5.15193}, {105.48, "Field Reading"=5.15141}, {105.519, "Field Reading"=5.15141}, {105.579, "Field Reading"=5.15088}, {105.621, "Field Reading"=5.15088}, {105.68, "Field Reading"=5.15046}, {105.719, "Field Reading"=5.15046}, {105.777, "Field Reading"=5.1501}, {105.815, "Field Reading"=5.1501}, {105.853, "Field Reading"=5.14962}, {105.908, "Field Reading"=5.14962}, {105.946, "Field Reading"=5.14931}, {106.007, "Field Reading"=5.14931}, {106.046, "Field Reading"=5.14915}, {106.108, "Field Reading"=5.14915}, {106.148, "Field Reading"=5.14889}, {106.205, "Field Reading"=5.14889}, {106.244, "Field Reading"=5.14889}, {106.294, "Field Reading"=5.14863}, {106.332, "Field Reading"=5.14863}, {106.393, "Field Reading"=5.14852}, {106.434, "Field Reading"=5.14852}, {106.494, "Field Reading"=5.14847}, {106.532, "Field Reading"=5.14847}, {106.579, "Field Reading"=5.14826}, {106.617, "Field Reading"=5.14826}, {106.675, "Field Reading"=5.1481}, {106.714, "Field Reading"=5.1481}, {106.775, "Field Reading"=5.14795}, {106.813, "Field Reading"=5.14795}, {106.852, "Field Reading"=5.14779}, {106.906, "Field Reading"=5.14779}, {106.946, "Field Reading"=5.14779}, {106.994, "Field Reading"=5.14748}, {107.035, "Field Reading"=5.14748}, {107.094, "Field Reading"=5.14727}, {107.133, "Field Reading"=5.14727}, {107.18, "Field Reading"=5.14685}, {107.218, "Field Reading"=5.14685}, {107.276, "Field Reading"=5.14659}, {107.315, "Field Reading"=5.14659}, {107.375, "Field Reading"=5.14643}, {107.415, "Field Reading"=5.14643}, {107.476, "Field Reading"=5.14648}, {107.516, "Field Reading"=5.14648}, {107.575, "Field Reading"=5.14659}, {107.614, "Field Reading"=5.14659}, {107.652, "Field Reading"=5.14659}, {107.707, "Field Reading"=5.14659}, {107.746, "Field Reading"=5.14664}, {107.808, "Field Reading"=5.14664}, {107.847, "Field Reading"=5.14664}, {107.907, "Field Reading"=5.14664}, {107.949, "Field Reading"=5.1468}, {108.008, "Field Reading"=5.1468}, {108.046, "Field Reading"=5.14664}, {108.107, "Field Reading"=5.14664}, {108.148, "Field Reading"=5.14638}, {108.206, "Field Reading"=5.14638}, {108.246, "Field Reading"=5.14596}, {108.308, "Field Reading"=5.14596}, {108.347, "Field Reading"=5.14543}, {108.406, "Field Reading"=5.14543}, {108.446, "Field Reading"=5.14543}, {108.496, "Field Reading"=5.1447}, {108.535, "Field Reading"=5.1447}, {108.594, "Field Reading"=5.14407}, {108.632, "Field Reading"=5.14407}, {108.682, "Field Reading"=5.1436}, {108.721, "Field Reading"=5.1436}, {108.779, "Field Reading"=5.14307}, {108.818, "Field Reading"=5.14307}, {108.882, "Field Reading"=5.14281}, {108.921, "Field Reading"=5.14281}, {108.98, "Field Reading"=5.14271}, {109.02, "Field Reading"=5.14271}, {109.081, "Field Reading"=5.1426}, {109.121, "Field Reading"=5.1426}, {109.18, "Field Reading"=5.14266}, {109.22, "Field Reading"=5.14266}, {109.281, "Field Reading"=5.1426}, {109.321, "Field Reading"=5.1426}, {109.38, "Field Reading"=5.14239}, {109.418, "Field Reading"=5.14239}, {109.476, "Field Reading"=5.14208}, {109.514, "Field Reading"=5.14208}, {109.575, "Field Reading"=5.14176}, {109.613, "Field Reading"=5.14176}, {109.652, "Field Reading"=5.14129}, {109.711, "Field Reading"=5.14129}, {109.751, "Field Reading"=5.14056}, {109.807, "Field Reading"=5.14056}, {109.846, "Field Reading"=5.14056}, {109.895, "Field Reading"=5.13988}, {109.934, "Field Reading"=5.13988}, {109.981, "Field Reading"=5.13904}, {110.019, "Field Reading"=5.13904}, {110.078, "Field Reading"=5.13841}, {110.121, "Field Reading"=5.13841}, {110.178, "Field Reading"=5.13804}, {110.218, "Field Reading"=5.13804}, {110.276, "Field Reading"=5.13773}, {110.316, "Field Reading"=5.13773}, {110.375, "Field Reading"=5.13752}, {110.414, "Field Reading"=5.13752}, {110.476, "Field Reading"=5.13731}, {110.515, "Field Reading"=5.13731}, {110.575, "Field Reading"=5.13705}, {110.613, "Field Reading"=5.13705}, {110.653, "Field Reading"=5.13673}, {110.707, "Field Reading"=5.13673}, {110.749, "Field Reading"=5.13652}, {110.807, "Field Reading"=5.13652}, {110.848, "Field Reading"=5.13631}, {110.907, "Field Reading"=5.13631}, {110.948, "Field Reading"=5.136}, {111.008, "Field Reading"=5.136}, {111.048, "Field Reading"=5.13574}, {111.107, "Field Reading"=5.13574}, {111.148, "Field Reading"=5.13558}, {111.207, "Field Reading"=5.13558}, {111.246, "Field Reading"=5.13558}, {111.296, "Field Reading"=5.13548}, {111.334, "Field Reading"=5.13548}, {111.394, "Field Reading"=5.13548}, {111.433, "Field Reading"=5.13548}, {111.482, "Field Reading"=5.13569}, {111.521, "Field Reading"=5.13569}, {111.581, "Field Reading"=5.13626}, {111.621, "Field Reading"=5.13626}, {111.681, "Field Reading"=5.13663}, {111.719, "Field Reading"=5.13663}, {111.78, "Field Reading"=5.13694}, {111.819, "Field Reading"=5.13694}, {111.879, "Field Reading"=5.13715}, {111.918, "Field Reading"=5.13715}, {111.976, "Field Reading"=5.13726}, {112.015, "Field Reading"=5.13726}, {112.054, "Field Reading"=5.13741}, {112.109, "Field Reading"=5.13741}, {112.148, "Field Reading"=5.13762}, {112.207, "Field Reading"=5.13762}, {112.246, "Field Reading"=5.13762}, {112.297, "Field Reading"=5.13773}, {112.336, "Field Reading"=5.13773}, {112.395, "Field Reading"=5.13736}, {112.434, "Field Reading"=5.13736}, {112.497, "Field Reading"=5.13726}, {112.535, "Field Reading"=5.13726}, {112.593, "Field Reading"=5.13715}, {112.633, "Field Reading"=5.13715}, {112.685, "Field Reading"=5.13694}, {112.723, "Field Reading"=5.13694}, {112.78, "Field Reading"=5.13652}, {112.82, "Field Reading"=5.13652}, {112.879, "Field Reading"=5.13605}, {112.917, "Field Reading"=5.13605}, {112.976, "Field Reading"=5.13553}, {113.014, "Field Reading"=5.13553}, {113.077, "Field Reading"=5.13474}, {113.117, "Field Reading"=5.13474}, {113.176, "Field Reading"=5.13385}, {113.215, "Field Reading"=5.13385}, {113.254, "Field Reading"=5.13296}, {113.307, "Field Reading"=5.13296}, {113.349, "Field Reading"=5.13207}, {113.407, "Field Reading"=5.13207}, {113.447, "Field Reading"=5.13207}, {113.497, "Field Reading"=5.13123}, {113.536, "Field Reading"=5.13123}, {113.595, "Field Reading"=5.13076}, {113.636, "Field Reading"=5.13076}, {113.695, "Field Reading"=5.13029}, {113.733, "Field Reading"=5.13029}, {113.781, "Field Reading"=5.12982}, {113.822, "Field Reading"=5.12982}, {113.88, "Field Reading"=5.1295}, {113.918, "Field Reading"=5.1295}, {113.977, "Field Reading"=5.12934}, {114.017, "Field Reading"=5.12934}, {114.055, "Field Reading"=5.12898}, {114.108, "Field Reading"=5.12898}, {114.148, "Field Reading"=5.12851}, {114.207, "Field Reading"=5.12851}, {114.246, "Field Reading"=5.12851}, {114.295, "Field Reading"=5.12804}, {114.336, "Field Reading"=5.12804}, {114.395, "Field Reading"=5.12714}, {114.435, "Field Reading"=5.12714}, {114.496, "Field Reading"=5.12599}, {114.535, "Field Reading"=5.12599}, {114.595, "Field Reading"=5.12489}, {114.633, "Field Reading"=5.12489}, {114.683, "Field Reading"=5.12384}, {114.721, "Field Reading"=5.12384}, {114.779, "Field Reading"=5.123}, {114.82, "Field Reading"=5.123}, {114.879, "Field Reading"=5.12222}, {114.918, "Field Reading"=5.12222}, {114.977, "Field Reading"=5.12143}, {115.019, "Field Reading"=5.12143}, {115.078, "Field Reading"=5.12075}, {115.119, "Field Reading"=5.12075}, {115.178, "Field Reading"=5.12002}, {115.216, "Field Reading"=5.12002}, {115.256, "Field Reading"=5.11949}, {115.309, "Field Reading"=5.11949}, {115.348, "Field Reading"=5.11949}, {115.395, "Field Reading"=5.11881}, {115.434, "Field Reading"=5.11881}, {115.496, "Field Reading"=5.11824}, {115.535, "Field Reading"=5.11824}, {115.595, "Field Reading"=5.1175}, {115.635, "Field Reading"=5.1175}, {115.682, "Field Reading"=5.11682}, {115.721, "Field Reading"=5.11682}, {115.778, "Field Reading"=5.11624}, {115.819, "Field Reading"=5.11624}, {115.878, "Field Reading"=5.11577}, {115.916, "Field Reading"=5.11577}, {115.976, "Field Reading"=5.11546}, {116.016, "Field Reading"=5.11546}, {116.055, "Field Reading"=5.11525}, {116.11, "Field Reading"=5.11525}, {116.148, "Field Reading"=5.11493}, {116.207, "Field Reading"=5.11493}, {116.247, "Field Reading"=5.11493}, {116.297, "Field Reading"=5.11473}, {116.336, "Field Reading"=5.11473}, {116.395, "Field Reading"=5.11467}, {116.436, "Field Reading"=5.11467}, {116.497, "Field Reading"=5.11462}, {116.538, "Field Reading"=5.11462}, {116.595, "Field Reading"=5.11457}, {116.635, "Field Reading"=5.11457}, {116.684, "Field Reading"=5.11441}, {116.723, "Field Reading"=5.11441}, {116.782, "Field Reading"=5.11441}, {116.82, "Field Reading"=5.11441}, {116.879, "Field Reading"=5.11425}, {116.918, "Field Reading"=5.11425}, {116.978, "Field Reading"=5.1142}, {117.017, "Field Reading"=5.1142}, {117.056, "Field Reading"=5.11383}, {117.109, "Field Reading"=5.11383}, {117.148, "Field Reading"=5.11383}, {117.196, "Field Reading"=5.11326}, {117.235, "Field Reading"=5.11326}, {117.296, "Field Reading"=5.11258}, {117.335, "Field Reading"=5.11258}, {117.383, "Field Reading"=5.11184}, {117.422, "Field Reading"=5.11184}, {117.48, "Field Reading"=5.11121}, {117.52, "Field Reading"=5.11121}, {117.578, "Field Reading"=5.11053}, {117.618, "Field Reading"=5.11053}, {117.656, "Field Reading"=5.10964}, {117.711, "Field Reading"=5.10964}, {117.75, "Field Reading"=5.10886}, {117.808, "Field Reading"=5.10886}, {117.846, "Field Reading"=5.10886}, {117.898, "Field Reading"=5.10812}, {117.937, "Field Reading"=5.10812}, {117.996, "Field Reading"=5.10744}, {118.036, "Field Reading"=5.10744}, {118.097, "Field Reading"=5.10686}, {118.137, "Field Reading"=5.10686}, {118.196, "Field Reading"=5.10608}, {118.235, "Field Reading"=5.10608}, {118.284, "Field Reading"=5.10498}, {118.324, "Field Reading"=5.10498}, {118.382, "Field Reading"=5.10377}, {118.422, "Field Reading"=5.10377}, {118.483, "Field Reading"=5.10252}, {118.522, "Field Reading"=5.10252}, {118.58, "Field Reading"=5.10094}, {118.62, "Field Reading"=5.10094}, {118.679, "Field Reading"=5.09953}, {118.72, "Field Reading"=5.09953}, {118.779, "Field Reading"=5.09801}, {118.818, "Field Reading"=5.09801}, {118.878, "Field Reading"=5.09654}, {118.917, "Field Reading"=5.09654}, {118.956, "Field Reading"=5.09539}, {119.011, "Field Reading"=5.09539}, {119.051, "Field Reading"=5.09429}, {119.109, "Field Reading"=5.09429}, {119.148, "Field Reading"=5.09429}, {119.198, "Field Reading"=5.09329}, {119.238, "Field Reading"=5.09329}, {119.297, "Field Reading"=5.0924}, {119.336, "Field Reading"=5.0924}, {119.383, "Field Reading"=5.09183}, {119.422, "Field Reading"=5.09183}, {119.481, "Field Reading"=5.09099}, {119.519, "Field Reading"=5.09099}, {119.578, "Field Reading"=5.09036}, {119.617, "Field Reading"=5.09036}, {119.655, "Field Reading"=5.08973}, {119.712, "Field Reading"=5.08973}, {119.75, "Field Reading"=5.0891}, {119.808, "Field Reading"=5.0891}, {119.847, "Field Reading"=5.0891}, {119.897, "Field Reading"=5.08863}, {119.938, "Field Reading"=5.08863}, {119.996, "Field Reading"=5.08816}, {120.034, "Field Reading"=5.08816}, {120.084, "Field Reading"=5.08795}, {120.125, "Field Reading"=5.08795}, {120.183, "Field Reading"=5.08774}, {120.221, "Field Reading"=5.08774}, {120.281, "Field Reading"=5.08769}, {120.321, "Field Reading"=5.08769}, {120.379, "Field Reading"=5.08732}, {120.419, "Field Reading"=5.08732}, {120.479, "Field Reading"=5.08685}, {120.519, "Field Reading"=5.08685}, {120.578, "Field Reading"=5.08617}, {120.618, "Field Reading"=5.08617}, {120.679, "Field Reading"=5.08533}, {120.717, "Field Reading"=5.08533}, {120.756, "Field Reading"=5.08465}, {120.809, "Field Reading"=5.08465}, {120.848, "Field Reading"=5.08465}, {120.898, "Field Reading"=5.0837}, {120.936, "Field Reading"=5.0837}, {120.984, "Field Reading"=5.08281}, {121.022, "Field Reading"=5.08281}, {121.081, "Field Reading"=5.08203}, {121.121, "Field Reading"=5.08203}, {121.179, "Field Reading"=5.0815}, {121.217, "Field Reading"=5.0815}, {121.257, "Field Reading"=5.08119}, {121.31, "Field Reading"=5.08119}, {121.349, "Field Reading"=5.08119}, {121.399, "Field Reading"=5.08119}, {121.438, "Field Reading"=5.08119}, {121.485, "Field Reading"=5.08124}, {121.526, "Field Reading"=5.08124}, {121.583, "Field Reading"=5.08119}, {121.621, "Field Reading"=5.08119}, {121.68, "Field Reading"=5.08124}, {121.72, "Field Reading"=5.08124}, {121.778, "Field Reading"=5.08129}, {121.817, "Field Reading"=5.08129}, {121.856, "Field Reading"=5.08145}, {121.911, "Field Reading"=5.08145}, {121.953, "Field Reading"=5.08155}, {122.01, "Field Reading"=5.08155}, {122.049, "Field Reading"=5.08155}, {122.098, "Field Reading"=5.08145}, {122.14, "Field Reading"=5.08145}, {122.197, "Field Reading"=5.08135}, {122.238, "Field Reading"=5.08135}, {122.297, "Field Reading"=5.08108}, {122.337, "Field Reading"=5.08108}, {122.398, "Field Reading"=5.08072}, {122.438, "Field Reading"=5.08072}, {122.498, "Field Reading"=5.08024}, {122.536, "Field Reading"=5.08024}, {122.597, "Field Reading"=5.07972}, {122.637, "Field Reading"=5.07972}, {122.686, "Field Reading"=5.07904}, {122.727, "Field Reading"=5.07904}, {122.785, "Field Reading"=5.07831}, {122.824, "Field Reading"=5.07831}, {122.884, "Field Reading"=5.07757}, {122.923, "Field Reading"=5.07757}, {122.984, "Field Reading"=5.07679}, {123.023, "Field Reading"=5.07679}, {123.082, "Field Reading"=5.07626}, {123.12, "Field Reading"=5.07626}, {123.178, "Field Reading"=5.07579}, {123.218, "Field Reading"=5.07579}, {123.279, "Field Reading"=5.07569}, {123.32, "Field Reading"=5.07569}, {123.379, "Field Reading"=5.07563}, {123.418, "Field Reading"=5.07563}, {123.457, "Field Reading"=5.07553}, {123.512, "Field Reading"=5.07553}, {123.553, "Field Reading"=5.07563}, {123.611, "Field Reading"=5.07563}, {123.652, "Field Reading"=5.07569}, {123.71, "Field Reading"=5.07569}, {123.75, "Field Reading"=5.07553}, {123.811, "Field Reading"=5.07553}, {123.849, "Field Reading"=5.07553}, {123.9, "Field Reading"=5.07542}, {123.938, "Field Reading"=5.07542}, {123.997, "Field Reading"=5.07521}, {124.035, "Field Reading"=5.07521}, {124.085, "Field Reading"=5.0749}, {124.125, "Field Reading"=5.0749}, {124.184, "Field Reading"=5.07464}, {124.225, "Field Reading"=5.07464}, {124.285, "Field Reading"=5.07443}, {124.324, "Field Reading"=5.07443}, {124.381, "Field Reading"=5.07401}, {124.421, "Field Reading"=5.07401}, {124.48, "Field Reading"=5.07364}, {124.521, "Field Reading"=5.07364}, {124.579, "Field Reading"=5.07333}, {124.617, "Field Reading"=5.07333}, {124.658, "Field Reading"=5.07301}, {124.711, "Field Reading"=5.07301}, {124.75, "Field Reading"=5.07301}, {124.798, "Field Reading"=5.07286}, {124.837, "Field Reading"=5.07286}, {124.898, "Field Reading"=5.07259}, {124.937, "Field Reading"=5.07259}, {124.984, "Field Reading"=5.07228}, {125.024, "Field Reading"=5.07228}, {125.083, "Field Reading"=5.07181}, {125.122, "Field Reading"=5.07181}, {125.18, "Field Reading"=5.07155}, {125.22, "Field Reading"=5.07155}, {125.28, "Field Reading"=5.07139}, {125.321, "Field Reading"=5.07139}, {125.379, "Field Reading"=5.07139}, {125.419, "Field Reading"=5.07139}, {125.48, "Field Reading"=5.07128}, {125.52, "Field Reading"=5.07128}, {125.579, "Field Reading"=5.07113}, {125.621, "Field Reading"=5.07113}, {125.681, "Field Reading"=5.07092}, {125.719, "Field Reading"=5.07092}, {125.779, "Field Reading"=5.07081}, {125.819, "Field Reading"=5.07081}, {125.881, "Field Reading"=5.07086}, {125.92, "Field Reading"=5.07086}, {125.958, "Field Reading"=5.07086}, {126.011, "Field Reading"=5.07086}, {126.051, "Field Reading"=5.07065}, {126.114, "Field Reading"=5.07065}, {126.152, "Field Reading"=5.07045}, {126.211, "Field Reading"=5.07045}, {126.25, "Field Reading"=5.07045}, {126.301, "Field Reading"=5.07034}, {126.34, "Field Reading"=5.07034}, {126.399, "Field Reading"=5.07024}, {126.438, "Field Reading"=5.07024}, {126.485, "Field Reading"=5.07029}, {126.526, "Field Reading"=5.07029}, {126.585, "Field Reading"=5.07029}, {126.625, "Field Reading"=5.07029}, {126.685, "Field Reading"=5.07018}, {126.725, "Field Reading"=5.07018}, {126.782, "Field Reading"=5.07003}, {126.82, "Field Reading"=5.07003}, {126.88, "Field Reading"=5.06984}, {126.921, "Field Reading"=5.06984}, {126.98, "Field Reading"=5.06953}, {127.019, "Field Reading"=5.06953}, {127.058, "Field Reading"=5.06916}, {127.113, "Field Reading"=5.06916}, {127.153, "Field Reading"=5.06895}, {127.211, "Field Reading"=5.06895}, {127.249, "Field Reading"=5.06895}, {127.3, "Field Reading"=5.06874}, {127.34, "Field Reading"=5.06874}, {127.397, "Field Reading"=5.06861}, {127.437, "Field Reading"=5.06861}, {127.485, "Field Reading"=5.06869}, {127.525, "Field Reading"=5.06869}, {127.584, "Field Reading"=5.06879}, {127.624, "Field Reading"=5.06879}, {127.687, "Field Reading"=5.06893}, {127.726, "Field Reading"=5.06893}, {127.785, "Field Reading"=5.06906}, {127.826, "Field Reading"=5.06906}, {127.887, "Field Reading"=5.06903}, {127.927, "Field Reading"=5.06903}, {127.985, "Field Reading"=5.06872}, {128.023, "Field Reading"=5.06872}, {128.082, "Field Reading"=5.06822}, {128.121, "Field Reading"=5.06822}, {128.18, "Field Reading"=5.06769}, {128.22, "Field Reading"=5.06769}, {128.281, "Field Reading"=5.06693}, {128.324, "Field Reading"=5.06693}, {128.381, "Field Reading"=5.06612}, {128.421, "Field Reading"=5.06612}, {128.481, "Field Reading"=5.06539}, {128.52, "Field Reading"=5.06539}, {128.558, "Field Reading"=5.06476}, {128.612, "Field Reading"=5.06476}, {128.65, "Field Reading"=5.06476}, {128.7, "Field Reading"=5.06418}, {128.739, "Field Reading"=5.06418}, {128.785, "Field Reading"=5.0635}, {128.824, "Field Reading"=5.0635}, {128.881, "Field Reading"=5.06287}, {128.921, "Field Reading"=5.06287}, {128.98, "Field Reading"=5.06201}, {129.019, "Field Reading"=5.06201}, {129.081, "Field Reading"=5.06133}, {129.119, "Field Reading"=5.06133}, {129.18, "Field Reading"=5.06075}, {129.218, "Field Reading"=5.06075}, {129.258, "Field Reading"=5.06041}, {129.314, "Field Reading"=5.06041}, {129.355, "Field Reading"=5.0602}, {129.412, "Field Reading"=5.0602}, {129.453, "Field Reading"=5.06017}, {129.514, "Field Reading"=5.06017}, {129.555, "Field Reading"=5.06041}, {129.611, "Field Reading"=5.06041}, {129.649, "Field Reading"=5.06041}, {129.7, "Field Reading"=5.06062}, {129.739, "Field Reading"=5.06062}, {129.8, "Field Reading"=5.06099}, {129.838, "Field Reading"=5.06099}, {129.9, "Field Reading"=5.06117}, {129.939, "Field Reading"=5.06117}, {129.987, "Field Reading"=5.06127}, {130.027, "Field Reading"=5.06127}, {130.086, "Field Reading"=5.06104}, {130.126, "Field Reading"=5.06104}, {130.185, "Field Reading"=5.06051}, {130.223, "Field Reading"=5.06051}, {130.282, "Field Reading"=5.05983}, {130.32, "Field Reading"=5.05983}, {130.38, "Field Reading"=5.05913}, {130.418, "Field Reading"=5.05913}, {130.457, "Field Reading"=5.0586}, {130.512, "Field Reading"=5.0586}, {130.552, "Field Reading"=5.0586}, {130.6, "Field Reading"=5.05787}, {130.64, "Field Reading"=5.05787}, {130.7, "Field Reading"=5.0574}, {130.743, "Field Reading"=5.0574}, {130.799, "Field Reading"=5.05698}, {130.839, "Field Reading"=5.05698}, {130.888, "Field Reading"=5.05656}, {130.929, "Field Reading"=5.05656}, {130.985, "Field Reading"=5.05645}, {131.023, "Field Reading"=5.05645}, {131.081, "Field Reading"=5.05627}, {131.12, "Field Reading"=5.05627}, {131.158, "Field Reading"=5.05596}, {131.213, "Field Reading"=5.05596}, {131.252, "Field Reading"=5.05596}, {131.301, "Field Reading"=5.05567}, {131.339, "Field Reading"=5.05567}, {131.386, "Field Reading"=5.05554}, {131.425, "Field Reading"=5.05554}, {131.483, "Field Reading"=5.05496}, {131.523, "Field Reading"=5.05496}, {131.581, "Field Reading"=5.05451}, {131.62, "Field Reading"=5.05451}, {131.658, "Field Reading"=5.05407}, {131.715, "Field Reading"=5.05407}, {131.755, "Field Reading"=5.05339}, {131.814, "Field Reading"=5.05339}, {131.851, "Field Reading"=5.05339}, {131.901, "Field Reading"=5.05286}, {131.941, "Field Reading"=5.05286}, {132.0, "Field Reading"=5.05239}, {132.039, "Field Reading"=5.05239}, {132.087, "Field Reading"=5.052}, {132.128, "Field Reading"=5.052}, {132.187, "Field Reading"=5.05171}, {132.226, "Field Reading"=5.05171}, {132.287, "Field Reading"=5.05187}, {132.328, "Field Reading"=5.05187}, {132.387, "Field Reading"=5.05189}, {132.427, "Field Reading"=5.05189}, {132.488, "Field Reading"=5.05187}, {132.528, "Field Reading"=5.05187}, {132.587, "Field Reading"=5.05197}, {132.628, "Field Reading"=5.05197}, {132.687, "Field Reading"=5.05197}, {132.726, "Field Reading"=5.05197}, {132.783, "Field Reading"=5.052}, {132.821, "Field Reading"=5.052}, {132.86, "Field Reading"=5.05176}, {132.913, "Field Reading"=5.05176}, {132.951, "Field Reading"=5.05176}, {133.0, "Field Reading"=5.05153}, {133.038, "Field Reading"=5.05153}, {133.088, "Field Reading"=5.05108}, {133.127, "Field Reading"=5.05108}, {133.184, "Field Reading"=5.05061}, {133.224, "Field Reading"=5.05061}, {133.282, "Field Reading"=5.05017}, {133.322, "Field Reading"=5.05017}, {133.36, "Field Reading"=5.04975}, {133.414, "Field Reading"=5.04975}, {133.453, "Field Reading"=5.04951}, {133.513, "Field Reading"=5.04951}, {133.552, "Field Reading"=5.04951}, {133.6, "Field Reading"=5.04904}, {133.64, "Field Reading"=5.04904}, {133.701, "Field Reading"=5.04859}, {133.739, "Field Reading"=5.04859}, {133.787, "Field Reading"=5.0481}, {133.825, "Field Reading"=5.0481}, {133.887, "Field Reading"=5.04768}, {133.927, "Field Reading"=5.04768}, {133.983, "Field Reading"=5.0472}, {134.024, "Field Reading"=5.0472}, {134.083, "Field Reading"=5.04665}, {134.124, "Field Reading"=5.04665}, {134.182, "Field Reading"=5.04589}, {134.223, "Field Reading"=5.04589}, {134.282, "Field Reading"=5.04516}, {134.321, "Field Reading"=5.04516}, {134.36, "Field Reading"=5.04456}, {134.414, "Field Reading"=5.04456}, {134.453, "Field Reading"=5.04456}, {134.503, "Field Reading"=5.04409}, {134.542, "Field Reading"=5.04409}, {134.601, "Field Reading"=5.04346}, {134.64, "Field Reading"=5.04346}, {134.702, "Field Reading"=5.04291}, {134.742, "Field Reading"=5.04291}, {134.8, "Field Reading"=5.04223}, {134.84, "Field Reading"=5.04223}, {134.888, "Field Reading"=5.04173}, {134.926, "Field Reading"=5.04173}, {134.983, "Field Reading"=5.04157}, {135.023, "Field Reading"=5.04157}, {135.082, "Field Reading"=5.04147}, {135.125, "Field Reading"=5.04147}, {135.182, "Field Reading"=5.04113}, {135.222, "Field Reading"=5.04113}, {135.282, "Field Reading"=5.04079}, {135.323, "Field Reading"=5.04079}, {135.382, "Field Reading"=5.04047}, {135.421, "Field Reading"=5.04047}, {135.46, "Field Reading"=5.0401}, {135.515, "Field Reading"=5.0401}, {135.554, "Field Reading"=5.03976}, {135.612, "Field Reading"=5.03976}, {135.65, "Field Reading"=5.03976}, {135.702, "Field Reading"=5.03927}, {135.742, "Field Reading"=5.03927}, {135.8, "Field Reading"=5.03872}, {135.839, "Field Reading"=5.03872}, {135.888, "Field Reading"=5.03809}, {135.926, "Field Reading"=5.03809}, {135.983, "Field Reading"=5.03785}, {136.022, "Field Reading"=5.03785}, {136.083, "Field Reading"=5.03751}, {136.123, "Field Reading"=5.03751}, {136.16, "Field Reading"=5.03714}, {136.213, "Field Reading"=5.03714}, {136.251, "Field Reading"=5.03714}, {136.302, "Field Reading"=5.0368}, {136.34, "Field Reading"=5.0368}, {136.387, "Field Reading"=5.03672}, {136.427, "Field Reading"=5.03672}, {136.488, "Field Reading"=5.03662}, {136.528, "Field Reading"=5.03662}, {136.589, "Field Reading"=5.03625}, {136.628, "Field Reading"=5.03625}, {136.688, "Field Reading"=5.03594}, {136.726, "Field Reading"=5.03594}, {136.784, "Field Reading"=5.03541}, {136.823, "Field Reading"=5.03541}, {136.883, "Field Reading"=5.03497}, {136.922, "Field Reading"=5.03497}, {136.961, "Field Reading"=5.03439}, {137.014, "Field Reading"=5.03439}, {137.054, "Field Reading"=5.03382}, {137.114, "Field Reading"=5.03382}, {137.153, "Field Reading"=5.03382}, {137.203, "Field Reading"=5.03321}, {137.246, "Field Reading"=5.03321}, {137.303, "Field Reading"=5.0324}, {137.343, "Field Reading"=5.0324}, {137.402, "Field Reading"=5.03159}, {137.442, "Field Reading"=5.03159}, {137.501, "Field Reading"=5.0307}, {137.542, "Field Reading"=5.0307}, {137.601, "Field Reading"=5.03002}, {137.641, "Field Reading"=5.03002}, {137.688, "Field Reading"=5.02915}, {137.727, "Field Reading"=5.02915}, {137.788, "Field Reading"=5.02837}, {137.828, "Field Reading"=5.02837}, {137.889, "Field Reading"=5.02769}, {137.926, "Field Reading"=5.02769}, {137.984, "Field Reading"=5.02687}, {138.023, "Field Reading"=5.02687}, {138.083, "Field Reading"=5.02653}, {138.124, "Field Reading"=5.02653}, {138.182, "Field Reading"=5.02637}, {138.222, "Field Reading"=5.02637}, {138.261, "Field Reading"=5.02606}, {138.317, "Field Reading"=5.02606}, {138.358, "Field Reading"=5.02562}, {138.414, "Field Reading"=5.02562}, {138.454, "Field Reading"=5.02541}, {138.515, "Field Reading"=5.02541}, {138.554, "Field Reading"=5.02541}, {138.602, "Field Reading"=5.02527}, {138.644, "Field Reading"=5.02527}, {138.703, "Field Reading"=5.02512}, {138.742, "Field Reading"=5.02512}, {138.801, "Field Reading"=5.02506}, {138.839, "Field Reading"=5.02506}, {138.89, "Field Reading"=5.02472}, {138.93, "Field Reading"=5.02472}, {138.988, "Field Reading"=5.02446}, {139.028, "Field Reading"=5.02446}, {139.089, "Field Reading"=5.02428}, {139.129, "Field Reading"=5.02428}, {139.187, "Field Reading"=5.02394}, {139.225, "Field Reading"=5.02394}, {139.284, "Field Reading"=5.02341}, {139.322, "Field Reading"=5.02341}, {139.361, "Field Reading"=5.02273}, {139.415, "Field Reading"=5.02273}, {139.455, "Field Reading"=5.02216}, {139.515, "Field Reading"=5.02216}, {139.554, "Field Reading"=5.02158}, {139.614, "Field Reading"=5.02158}, {139.652, "Field Reading"=5.02158}, {139.704, "Field Reading"=5.02116}, {139.743, "Field Reading"=5.02116}, {139.802, "Field Reading"=5.02064}, {139.843, "Field Reading"=5.02064}, {139.902, "Field Reading"=5.02014}, {139.942, "Field Reading"=5.02014}, {140.0, "Field Reading"=5.01962}, {140.039, "Field Reading"=5.01962}, {140.089, "Field Reading"=5.0192}, {140.128, "Field Reading"=5.0192}, {140.188, "Field Reading"=5.01878}, {140.23, "Field Reading"=5.01878}, {140.289, "Field Reading"=5.01828}, {140.328, "Field Reading"=5.01828}, {140.389, "Field Reading"=5.01768}, {140.429, "Field Reading"=5.01768}, {140.489, "Field Reading"=5.01692}, {140.527, "Field Reading"=5.01692}, {140.585, "Field Reading"=5.01621}, {140.624, "Field Reading"=5.01621}, {140.685, "Field Reading"=5.01569}, {140.723, "Field Reading"=5.01569}, {140.761, "Field Reading"=5.01513}, {140.816, "Field Reading"=5.01513}, {140.854, "Field Reading"=5.01513}, {140.904, "Field Reading"=5.01451}, {140.945, "Field Reading"=5.01451}, {141.001, "Field Reading"=5.01409}, {141.041, "Field Reading"=5.01409}, {141.103, "Field Reading"=5.01375}, {141.142, "Field Reading"=5.01375}, {141.202, "Field Reading"=5.01354}, {141.241, "Field Reading"=5.01354}, {141.289, "Field Reading"=5.01314}, {141.328, "Field Reading"=5.01314}, {141.385, "Field Reading"=5.01267}, {141.423, "Field Reading"=5.01267}, {141.461, "Field Reading"=5.0121}, {141.516, "Field Reading"=5.0121}, {141.557, "Field Reading"=5.01181}, {141.614, "Field Reading"=5.01181}, {141.654, "Field Reading"=5.01181}, {141.703, "Field Reading"=5.01168}, {141.742, "Field Reading"=5.01168}, {141.802, "Field Reading"=5.0116}, {141.845, "Field Reading"=5.0116}, {141.902, "Field Reading"=5.01144}, {141.941, "Field Reading"=5.01144}, {142.003, "Field Reading"=5.01123}, {142.043, "Field Reading"=5.01123}, {142.102, "Field Reading"=5.01139}, {142.14, "Field Reading"=5.01139}, {142.188, "Field Reading"=5.01168}, {142.227, "Field Reading"=5.01168}, {142.287, "Field Reading"=5.01186}, {142.326, "Field Reading"=5.01186}, {142.384, "Field Reading"=5.0117}, {142.423, "Field Reading"=5.0117}, {142.484, "Field Reading"=5.01155}, {142.524, "Field Reading"=5.01155}, {142.584, "Field Reading"=5.01141}, {142.622, "Field Reading"=5.01141}, {142.661, "Field Reading"=5.01149}, {142.716, "Field Reading"=5.01149}, {142.755, "Field Reading"=5.01149}, {142.805, "Field Reading"=5.01157}, {142.842, "Field Reading"=5.01157}, {142.903, "Field Reading"=5.01152}, {142.942, "Field Reading"=5.01152}, {142.989, "Field Reading"=5.0112}, {143.028, "Field Reading"=5.0112}, {143.087, "Field Reading"=5.01099}, {143.125, "Field Reading"=5.01099}, {143.184, "Field Reading"=5.01086}, {143.222, "Field Reading"=5.01086}, {143.285, "Field Reading"=5.01065}, {143.325, "Field Reading"=5.01065}, {143.384, "Field Reading"=5.01018}, {143.425, "Field Reading"=5.01018}, {143.485, "Field Reading"=5.00942}, {143.526, "Field Reading"=5.00942}, {143.584, "Field Reading"=5.00864}, {143.622, "Field Reading"=5.00864}, {143.661, "Field Reading"=5.00769}, {143.718, "Field Reading"=5.00769}, {143.758, "Field Reading"=5.00699}, {143.815, "Field Reading"=5.00699}, {143.853, "Field Reading"=5.00699}, {143.903, "Field Reading"=5.00638}, {143.941, "Field Reading"=5.00638}, {143.989, "Field Reading"=5.00604}, {144.027, "Field Reading"=5.00604}, {144.086, "Field Reading"=5.00575}, {144.125, "Field Reading"=5.00575}, {144.184, "Field Reading"=5.00575}, {144.222, "Field Reading"=5.00575}, {144.262, "Field Reading"=5.00602}, {144.316, "Field Reading"=5.00602}, {144.355, "Field Reading"=5.00602}, {144.404, "Field Reading"=5.00638}, {144.443, "Field Reading"=5.00638}, {144.504, "Field Reading"=5.00678}, {144.543, "Field Reading"=5.00678}, {144.602, "Field Reading"=5.00693}, {144.642, "Field Reading"=5.00693}, {144.691, "Field Reading"=5.00704}, {144.731, "Field Reading"=5.00704}, {144.789, "Field Reading"=5.00701}, {144.829, "Field Reading"=5.00701}, {144.887, "Field Reading"=5.00704}, {144.926, "Field Reading"=5.00704}, {144.985, "Field Reading"=5.00696}, {145.025, "Field Reading"=5.00696}, {145.086, "Field Reading"=5.00654}, {145.125, "Field Reading"=5.00654}, {145.184, "Field Reading"=5.0061}, {145.222, "Field Reading"=5.0061}, {145.261, "Field Reading"=5.00581}, {145.316, "Field Reading"=5.00581}, {145.355, "Field Reading"=5.00581}, {145.405, "Field Reading"=5.0057}, {145.446, "Field Reading"=5.0057}, {145.504, "Field Reading"=5.0056}, {145.543, "Field Reading"=5.0056}, {145.589, "Field Reading"=5.00547}, {145.627, "Field Reading"=5.00547}, {145.686, "Field Reading"=5.00534}, {145.724, "Field Reading"=5.00534}, {145.763, "Field Reading"=5.00515}, {145.816, "Field Reading"=5.00515}, {145.856, "Field Reading"=5.00515}, {145.905, "Field Reading"=5.00515}, {145.946, "Field Reading"=5.00515}, {146.004, "Field Reading"=5.00507}, {146.044, "Field Reading"=5.00507}, {146.105, "Field Reading"=5.00479}, {146.145, "Field Reading"=5.00479}, {146.202, "Field Reading"=5.00465}, {146.242, "Field Reading"=5.00465}, {146.29, "Field Reading"=5.00444}, {146.329, "Field Reading"=5.00444}, {146.386, "Field Reading"=5.00426}, {146.426, "Field Reading"=5.00426}, {146.485, "Field Reading"=5.00408}, {146.524, "Field Reading"=5.00408}, {146.563, "Field Reading"=5.00376}, {146.617, "Field Reading"=5.00376}, {146.657, "Field Reading"=5.00337}, {146.717, "Field Reading"=5.00337}, {146.756, "Field Reading"=5.00293}, {146.817, "Field Reading"=5.00293}, {146.856, "Field Reading"=5.00264}, {146.916, "Field Reading"=5.00264}, {146.957, "Field Reading"=5.00217}, {147.016, "Field Reading"=5.00217}, {147.055, "Field Reading"=5.00217}, {147.105, "Field Reading"=5.00177}, {147.144, "Field Reading"=5.00177}, {147.203, "Field Reading"=5.00146}, {147.242, "Field Reading"=5.00146}, {147.291, "Field Reading"=5.00112}, {147.331, "Field Reading"=5.00112}, {147.391, "Field Reading"=5.0008}, {147.43, "Field Reading"=5.0008}, {147.49, "Field Reading"=5.00065}, {147.529, "Field Reading"=5.00065}, {147.587, "Field Reading"=5.0007}, {147.625, "Field Reading"=5.0007}, {147.686, "Field Reading"=5.00075}, {147.727, "Field Reading"=5.00075}, {147.784, "Field Reading"=5.00114}, {147.823, "Field Reading"=5.00114}, {147.863, "Field Reading"=5.00151}, {147.918, "Field Reading"=5.00151}, {147.957, "Field Reading"=5.00172}, {148.019, "Field Reading"=5.00172}, {148.058, "Field Reading"=5.00182}, {148.116, "Field Reading"=5.00182}, {148.156, "Field Reading"=5.00182}, {148.205, "Field Reading"=5.00193}, {148.245, "Field Reading"=5.00193}, {148.304, "Field Reading"=5.00219}, {148.342, "Field Reading"=5.00219}, {148.39, "Field Reading"=5.00235}, {148.428, "Field Reading"=5.00235}, {148.487, "Field Reading"=5.00227}, {148.527, "Field Reading"=5.00227}, {148.587, "Field Reading"=5.0018}, {148.627, "Field Reading"=5.0018}, {148.687, "Field Reading"=5.00109}, {148.727, "Field Reading"=5.00109}, {148.785, "Field Reading"=5.00036}, {148.823, "Field Reading"=5.00036}, {148.863, "Field Reading"=4.99983}, {148.918, "Field Reading"=4.99983}, {148.957, "Field Reading"=4.9992}, {149.016, "Field Reading"=4.9992}, {149.054, "Field Reading"=4.9992}, {149.105, "Field Reading"=4.99831}, {149.145, "Field Reading"=4.99831}, {149.203, "Field Reading"=4.99732}, {149.244, "Field Reading"=4.99732}, {149.293, "Field Reading"=4.99638}, {149.332, "Field Reading"=4.99638}, {149.39, "Field Reading"=4.99588}, {149.43, "Field Reading"=4.99588}, {149.492, "Field Reading"=4.99541}, {149.531, "Field Reading"=4.99541}, {149.59, "Field Reading"=4.99504}, {149.628, "Field Reading"=4.99504}, {149.687, "Field Reading"=4.9942}, {149.727, "Field Reading"=4.9942}, {149.786, "Field Reading"=4.99349}, {149.826, "Field Reading"=4.99349}, {149.887, "Field Reading"=4.99276}, {149.926, "Field Reading"=4.99276}, {149.986, "Field Reading"=4.99221}, {150.024, "Field Reading"=4.99221}, {150.064, "Field Reading"=4.99168}, {150.118, "Field Reading"=4.99168}, {150.156, "Field Reading"=4.99168}, {150.206, "Field Reading"=4.99095}, {150.245, "Field Reading"=4.99095}, {150.306, "Field Reading"=4.99022}, {150.344, "Field Reading"=4.99022}, {150.403, "Field Reading"=4.98954}, {150.444, "Field Reading"=4.98954}, {150.505, "Field Reading"=4.98938}, {150.543, "Field Reading"=4.98938}, {150.59, "Field Reading"=4.9892}, {150.63, "Field Reading"=4.9892}, {150.693, "Field Reading"=4.98946}, {150.731, "Field Reading"=4.98946}, {150.788, "Field Reading"=4.98961}, {150.828, "Field Reading"=4.98961}, {150.887, "Field Reading"=4.98956}, {150.926, "Field Reading"=4.98956}, {150.986, "Field Reading"=4.98938}, {151.026, "Field Reading"=4.98938}, {151.087, "Field Reading"=4.98933}, {151.126, "Field Reading"=4.98933}, {151.186, "Field Reading"=4.98909}, {151.224, "Field Reading"=4.98909}, {151.265, "Field Reading"=4.98859}, {151.32, "Field Reading"=4.98859}, {151.361, "Field Reading"=4.98807}, {151.418, "Field Reading"=4.98807}, {151.457, "Field Reading"=4.98807}, {151.508, "Field Reading"=4.98726}, {151.546, "Field Reading"=4.98726}, {151.604, "Field Reading"=4.98639}, {151.646, "Field Reading"=4.98639}, {151.705, "Field Reading"=4.98555}, {151.744, "Field Reading"=4.98555}, {151.791, "Field Reading"=4.9849}, {151.83, "Field Reading"=4.9849}, {151.889, "Field Reading"=4.98409}, {151.93, "Field Reading"=4.98409}, {151.987, "Field Reading"=4.9833}, {152.026, "Field Reading"=4.9833}, {152.087, "Field Reading"=4.98251}, {152.125, "Field Reading"=4.98251}, {152.164, "Field Reading"=4.98178}, {152.218, "Field Reading"=4.98178}]
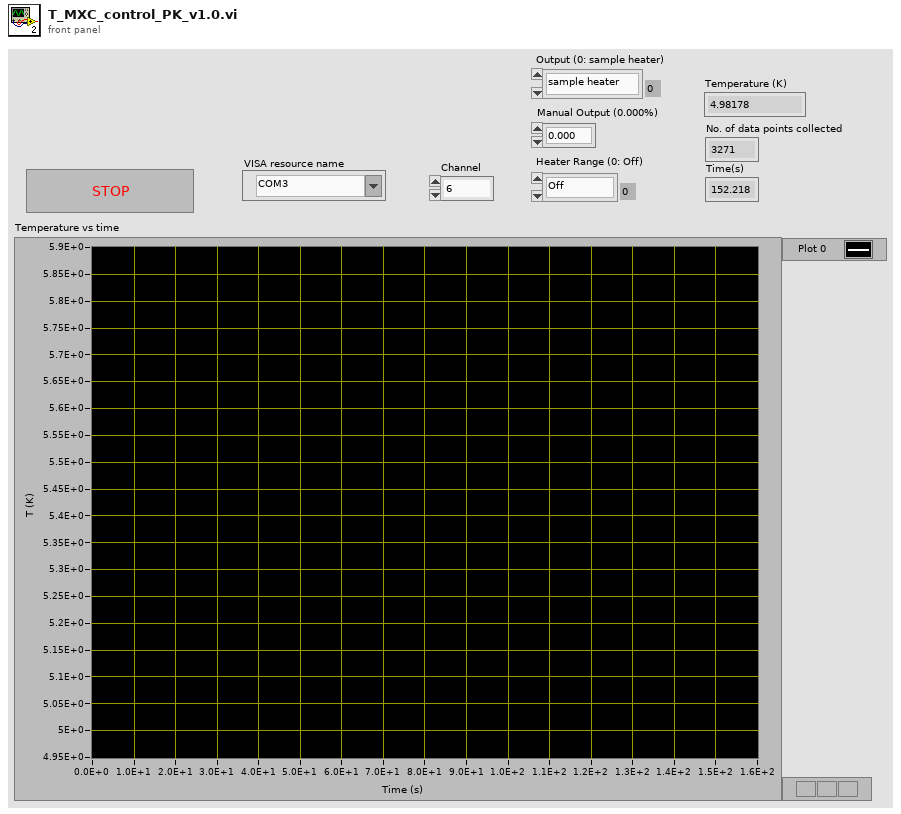
[diagram p1: front panel]
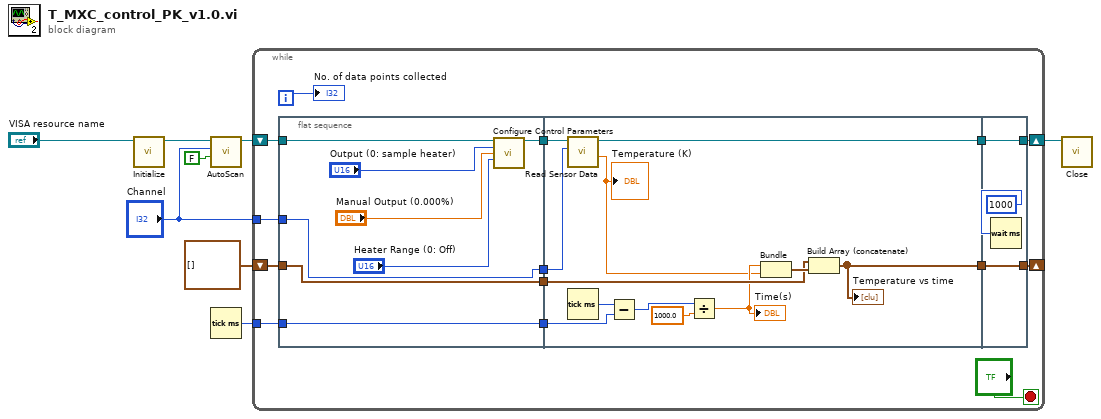
[diagram p0: block diagram]
diagram:
  n1 = call "Initialize.vi"("VISA resource name"="VISA resource name") -> ("VISA resource name out"=w4:refnum<visa-resource-name>)  [unwired: 9 in, 1 out]
  n2 = call "AutoScan.vi"("Autoscan (F: Off)"=FALSE, "Channel (1:1)"="Channel", "VISA resource name"=w4) -> ("VISA resource name out"=w5:refnum<visa-resource-name>)  [unwired: 7 in, 1 out]
  n3 = Tick Count (ms)() -> (millisecond timer value=w8:u32)
  n4 = while {
    tunnel: w8 -> [w20]
    shift-right: [w21] -> _
    shift-left: cluster{dbl, "Field Reading":dbl}[] [] -> [w22]
    shift-right: [w16] -> w2
    shift-left: w5 -> [w18]
    tunnel: "Channel" -> [w15]
    i -> [w17]
    stop <- "?" stop-if-true
    n5 = flat-sequence {
      tunnel: w15 -> [w28]
      tunnel: w18 -> [w26]
      tunnel: w20 -> [w29]
      tunnel: w22 -> [w30]
      tunnel: [w30] -> w14
      tunnel: [w29] -> w13
      tunnel: [w27] -> w12
      tunnel: [w28] -> w11
      tunnel: w14 -> [w41]
      tunnel: w13 -> [w38]
      tunnel: w12 -> [w33]
      tunnel: w11 -> [w31]
      tunnel: [w40] -> w10
      tunnel: [w32] -> w9
      tunnel: [w44] -> w16
      tunnel: [w45] -> w21
      tunnel: w10 -> [w45]
      tunnel: w9 -> [w44]
      frame #0 {
        n6 = call "Configure Control Parameters.vi"("VISA resource name"=w26, "Output (0: sample heater)"="Output (0: sample heater)", "Manual Output (0.000%)"="Manual Output (0.000%)", "Heater Range (0: Off)"="Heater Range (0: Off)") -> ("VISA resource name out"=w27:refnum<visa-resource-name>)  [unwired: 10 in, 1 out]
      }
      frame #1 {
        n7 = call "Read Sensor Data.vi"("Channel (1:1)"=w31, "VISA resource name"=w33) -> ("Kelvin Reading"=w34:dbl, "VISA resource name out"=w32:refnum<visa-resource-name>)  [unwired: 4 in, 4 out]
        "Temperature (K)" <- w34
        n8 = Tick Count (ms)() -> (millisecond timer value=w39:u32)
        n9 = Subtract(x=w39, y=w38) -> (x-y=w37:u32)
        n10 = Divide(x=w37, y=1000.0) -> (x/y=w35:dbl)
        "Time(s)" <- w35
        n11 = Bundle(w35, "Kelvin Reading"=w34) -> (w42:cluster{dbl, "Kelvin Reading":dbl})  [unwired: 1 in]
        n12 = Build Array (concatenate)(w41, w42) -> (w40:cluster{dbl, "Kelvin Reading":dbl}[])
        "Temperature vs time" <- w40
      }
      frame #2 {
        n13 = Wait (ms)(milliseconds to wait=1000) -> ()  [unwired: 1 out]
      }
    }
    "No. of data points collected" <- w17
  }
  n14 = call "Close.vi"("VISA resource name"=w2) -> ()  [unwired: 10 in, 1 out]
